vi "Sievert_auto.vi"() -> ()   [LabVIEW 2011]
uses:
  <vilib>/Utility/error.llb/DialogType.ctl
  <vilib>/DAQmx/write.llb/DAQmx Write (Digital Bool 1Line 1Point).vi
  <vilib>/Analysis/Matrix/Numeric/Conversions/Array To Matrix - RA.vi
  <vilib>/Analysis/Matrix/Numeric/Conversions/Matrix To Array - RM.vi
  <vilib>/DAQmx/create/channels.llb/DAQmx Create Channel (DO-Digital Output).vi
  <vilib>/DAQmx/miscellaneous.llb/DAQmx Fill In Error Info.vi
  <vilib>/Analysis/NI_AALPro.lvlib
  <vilib>/Analysis/Matrix/NI_Matrix.lvlib
  <vilib>/Analysis/NI_AALBase.lvlib
panel:
  in  "N fit patamar":i32=100
  in  "patamar milliseconds to wait":u32=500
  out "estagio 5":i32
  out "FIM":bool=TRUE
  out "limpo":i32
  in  "N fit":i32=5
  in  "Estagio auto":i32
  in  "ATM wait":u32
  in  "SET":i32
  in  "time subarray":dbl[](array[numeric])
  out "P cinetica mean 2":dbl format="%0.2f"
  out "T cinetica mean 3":dbl format="%0.2f"
  out "Time cinetica":dbl format="%0.2f"
  in  "T subarray 3":dbl[](array[numeric])
  in  "P T  index 2":i32
  in  "P subarray 2":dbl[](array[numeric])
  in  "Numeric":dbl=4.0
  in  "T subarray 2":dbl[](array[numeric])
  out "T cinetica mean 2":dbl format="%0.2f"
  out "P cinetica mean":dbl format="%0.2f"
  in  "P subarray":dbl[](array[numeric])
  in  "P T  index":i32
  out "T string":string
  out "P string":string
  out "path 2_cinetica":path
  out "Polynomial Coefficients 2":dbl[](array[numeric])
  out "Polynomial Coefficients":dbl[](array[numeric])
  in  "Count SET":i32=-1
  out "Set atual":i32
  out "mean pressure":dbl format="%.4p"
  out "Set number":i32
  in  "Tab Control":enum32{"Manual", "Automatico", "RLC - CDH2"}(tab)
  out "T":bool
  out "ZPf2":bool
  out "Pf2":bool
  out "Pit":bool
  out "ZPit":bool
  out "Camara":dbl(slide) scale=0.0..20.0 scale format="%#_3g"
  in  "Save manual":bool
  in  "Open Button":bool
  out "String 2":string
  in  "ATM":bool
  in  "Câmara":bool
  in  "Vácuo":bool
  in  "Entrada Gás":bool
  in  "Manual Ctrl":bool
  in  "stop":bool
  out "P-manual":dynamicdata(graph)
  in  "Clear":bool
  out "path":path
  in  "Nota":string
  in  "Sample name":string
  in  "File name":string
  out "Linear Model Graph":dbl[][](graph)
  out "Linear Model Graph 2":dbl[][](graph)
  in  "N to fit":i32=60
  out "N":i32
  out "Vácuo":bool
  out "Atm":bool
  out "Câmara":bool
  out "String_cinetica":string
  out "Vol Ref":dbl(slide) scale=0.0..50.0 scale format="%#_4f"
  out "Entrada gás":bool
  in  "Guardar\nCinetica":bool
  out "p fit":dbl format="%#_4g"
  out "T fit":dbl format="%#_4g"
  in  "Open Button 2":bool
  out "x >= y?":bool
  in  "seconds":dbl
  out "Elapsed Time (sec)":dbl format="%.1f"
  out "Boolean 3":bool
  out "String 3":string
  out "T 2":bool
  out "ZPit 2":bool
  out "Pit 2":bool
  out "Pf2 2":bool
  out "ZPf2 2":bool
  out "Camara 2":dbl(slide) scale=0.0..6.0 scale format="%#_3g"
  out "Vácuo 2":bool
  out "Atm 2":bool
  out "Câmara 2":bool
  out "Vol Ref 3":dbl(slide) scale=0.0..6.0 scale format="%#_4f"
  out "Entrada gás 2":bool
  in  "Auto Ctrl":bool
  in  "Play Button":bool
  out "time stamp":timestamp format="%<%.2X>T"
  out "Time (sec)":dbl format="%.1f"
  in  "clear":bool
  out "Automatico":dynamicdata(graph)
  out "Linear P":T1(graph)
  out "Linear T":T1(graph)
  out "Contador":i32
  in  "STOP Slope":dbl
  out "P slope":dbl
  out "slope":dbl format="%#_4g"
  out "P fit":dbl format="%#_4g"
  out "T fit":dbl format="%#_4g"
  out "x = y?":bool
  out "teste slope":i32
  in  "Set P auto":dbl
  in  "Step P":dbl=2.0
  in  "P_max":dbl=2.0
  in  "P_max camara":dbl=2.0
  out "Carga":bool=TRUE
  out "Descarga":bool
  out "String":string
  in  "P_min descarga":dbl
  in  "Boolean":bool
  in  "Array":dbl[](array[numeric])
  out "Boolean 2":bool
  out "Desc SET":i32
  in  "ZPf2 time":dbl=24.0
  in  "Ciclos":dbl
  out "Efetuados":dbl
  # "P vol ref"
  # "P Câmara"
  # "P vol ref"
  # "P Câmara"
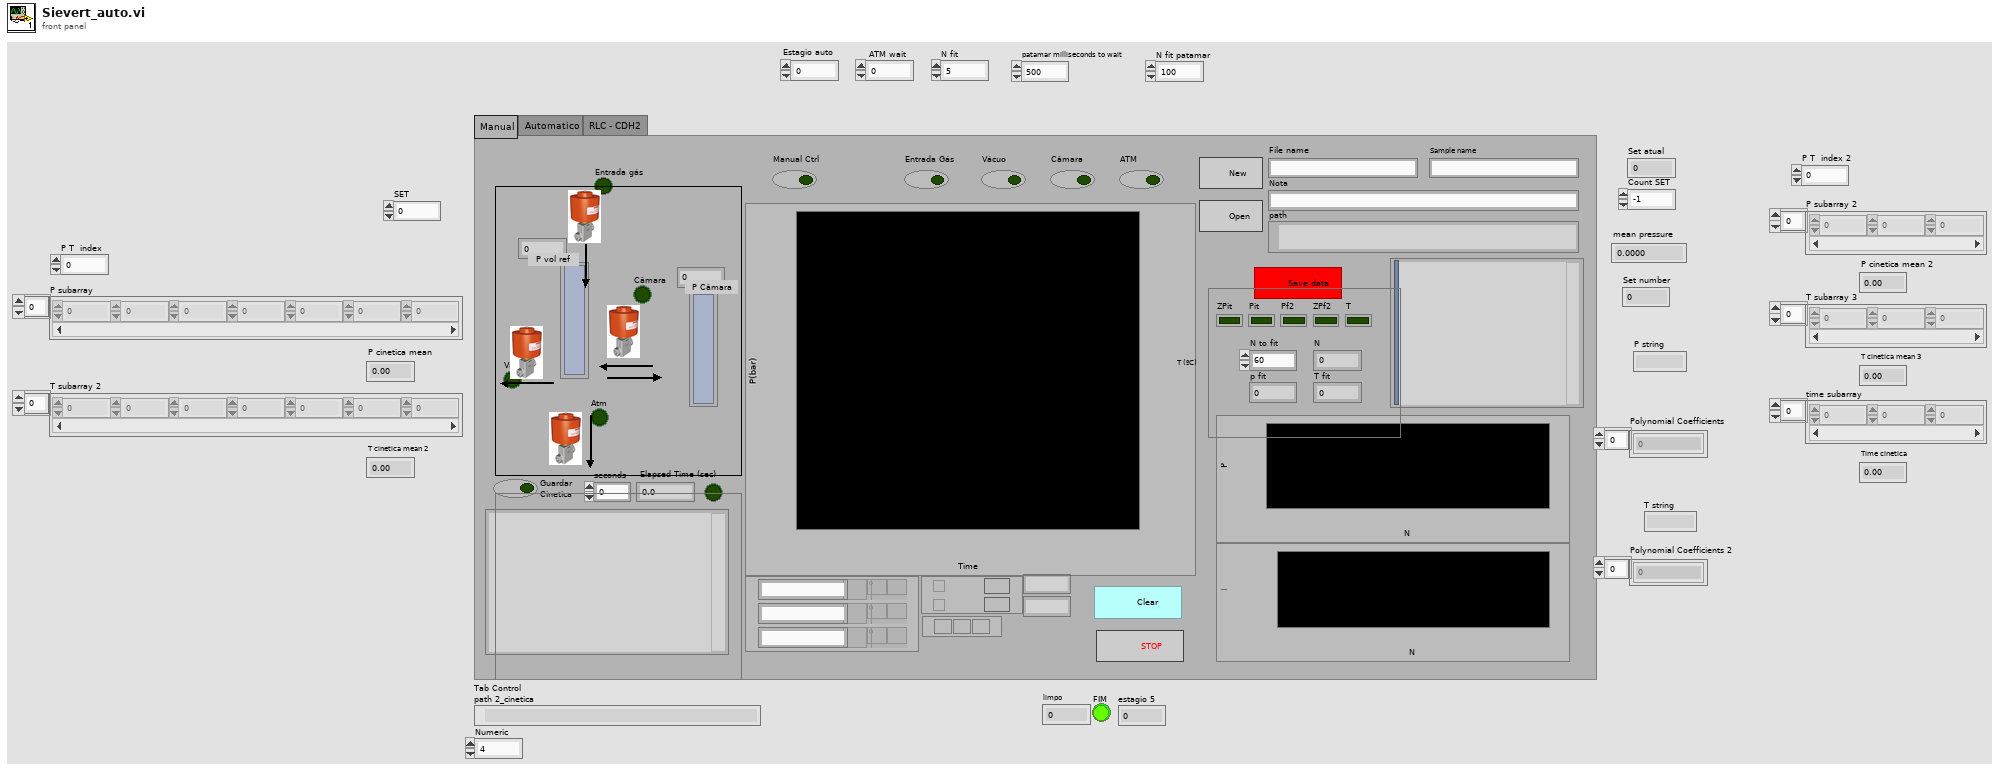
[diagram p1: front panel]
types:
  T1 = cluster{"Real 2D Array":dbl[], "Best Linear Fit":dbl[]}[]
  T2 = enum16{"open", "replace", "create", "open or create", "replace or create", "replace or create with confirmation"}
  T3 = typedef "NI_Matrix.lvlib/RealMatrix.ctl" = dbl[][]
  T4 = typedef "DialogType.ctl" = u16
  T5 = cluster{"Real 2D Array":dbl[], "Best Polynomial Fit":dbl[]}
  T6 = cluster{"Real 2D Array":dbl[], "Best Linear Fit":dbl[]}
  T7 = cluster{"Real 2D Array":dbl[], "Real 2D Array":dbl[]}
  T8 = cluster{"Real 2D Array":dbl[], "Best Polynomial Fit":dbl[]}[]
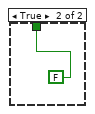
[diagram p2: hidden frame]
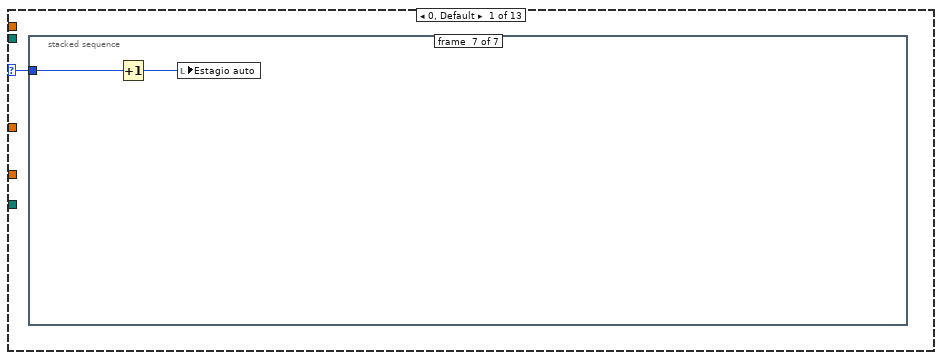
[diagram p5: hidden frame]
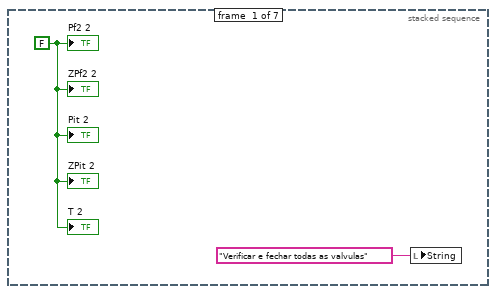
[diagram p6: hidden frame]
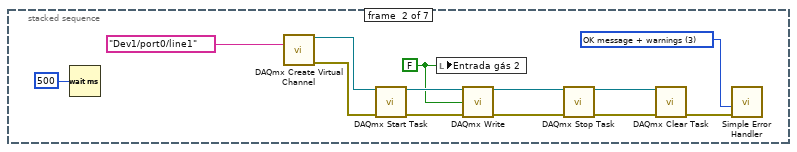
[diagram p7: hidden frame]
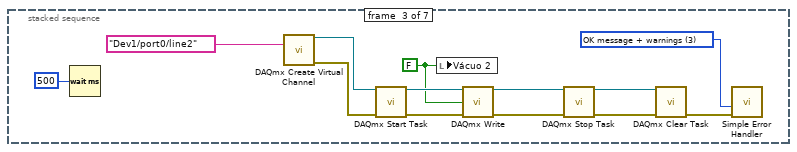
[diagram p8: hidden frame]
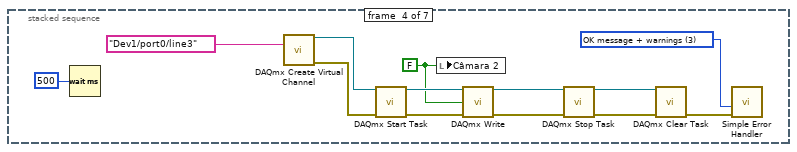
[diagram p9: hidden frame]
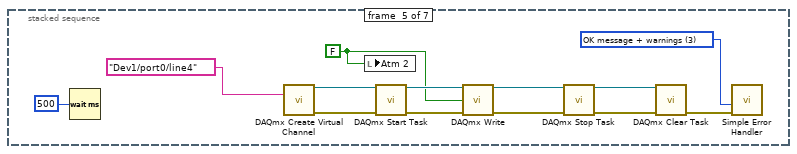
[diagram p10: hidden frame]
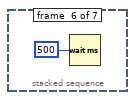
[diagram p11: hidden frame]
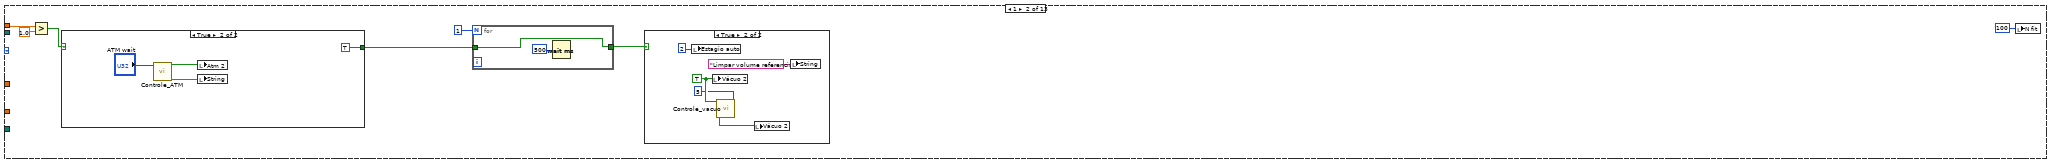
[diagram p12: hidden frame]
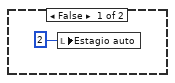
[diagram p13: hidden frame]
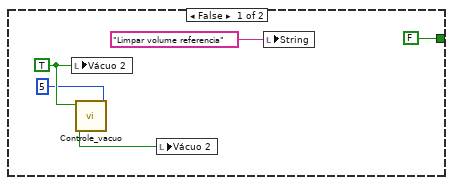
[diagram p14: hidden frame]
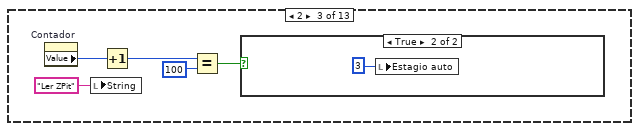
[diagram p15: hidden frame]
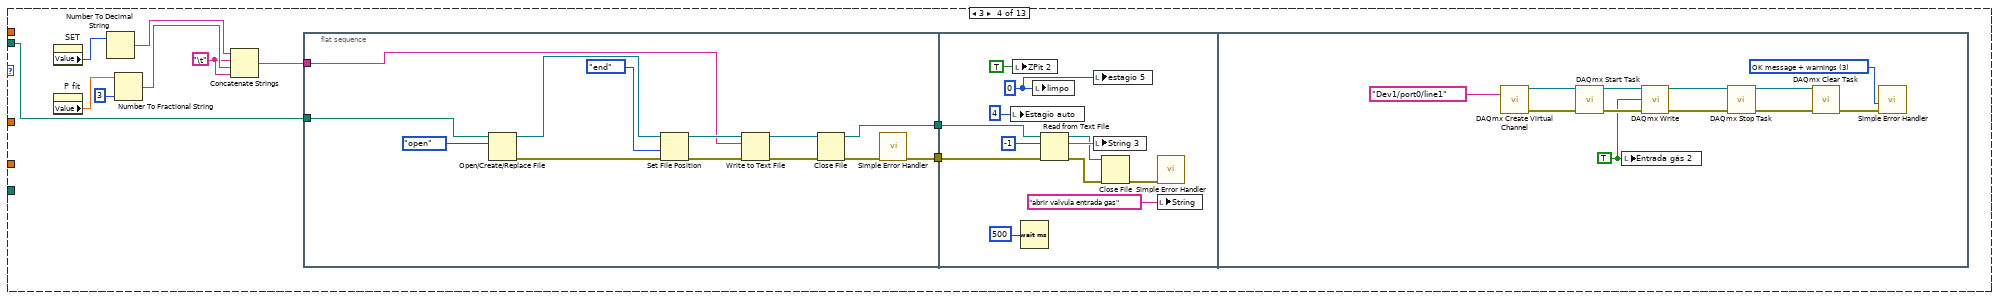
[diagram p17: hidden frame]
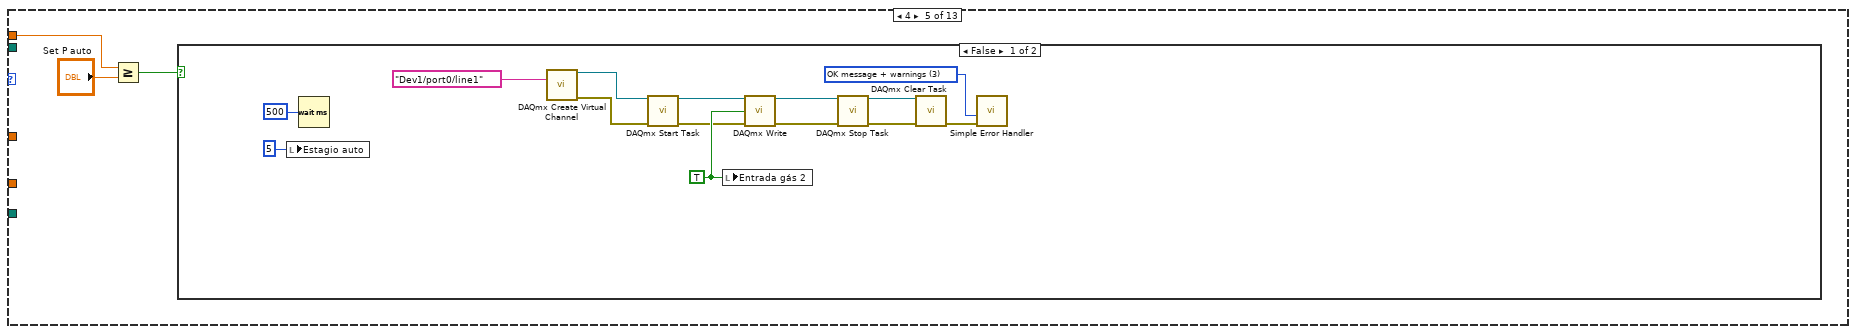
[diagram p18: hidden frame]
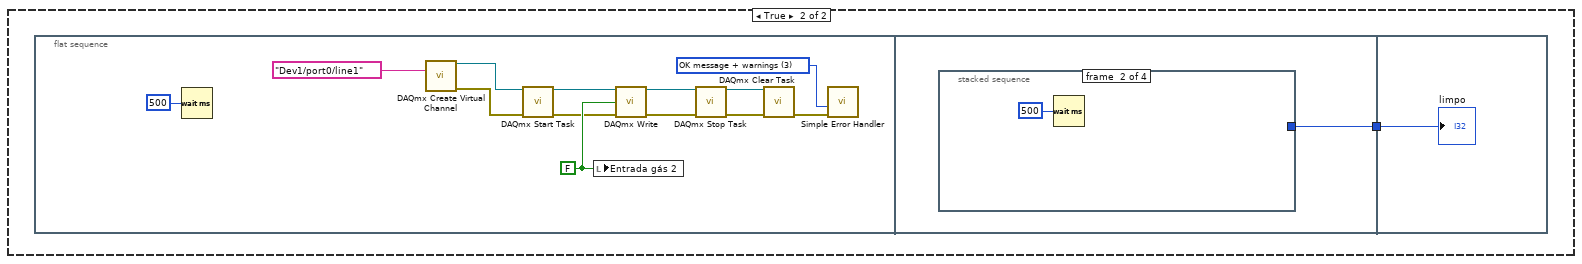
[diagram p19: hidden frame]
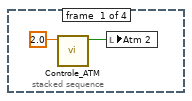
[diagram p20: hidden frame]
diagram:
  n1 = local write "P_min descarga"(0.025 ("P_min descarga")) -> ()
  n2 = local write "P_max camara"(25.0 ("P_max camara")) -> ()
  n3 = local write "Array"(dbl[] [0.5, 1.0, 2.0, 3.0, 4.0, 5.0, 6.0, 7.0, 8.0, 9.0, 10.0, 11.0, 12.0, 13.0, 14.0, 15.0, 16.0, 17.0, 18.0, 19.0, 20.0, 30.0, 40.0, 50.0, 60.0, 70.0] ("Array")) -> ()
  n4 = local write "Set P auto"(0.5 ("Set P auto")) -> ()
  n5 = local write "teste slope"(0 ("teste slope")) -> ()
  n6 = local write "Efetuados"(0.0 ("Efetuados")) -> ()
  n7 = local write "Desc SET"(0 ("Desc SET")) -> ()
  n8 = local write "P_max"(50.0 ("P_max")) -> ()
  n9 = local write "Ciclos"(0.0 ("Ciclos")) -> ()
  n10 = local write "Carga"(TRUE ("Carga")) -> ()
  n11 = local write "Descarga"(FALSE ("Descarga")) -> ()
  n12 = local write "estagio 5"(0 ("estagio 5")) -> ()
  n13 = local write "SET"(0 ("SET auto")) -> ()
  n14 = while {
    stop <- w28 stop-if-true
    n15 = case shown="False" "Auto Ctrl" {
      tunnel: [TRUE ("Auto Ctrl") FALSE ("Auto Ctrl")] -> w29
      frame False {
      }
      frame True {
      }
    }
    n16 = local write "Manual Ctrl"(w29) -> ()
    n17 = case shown="True" "Auto Ctrl" {
      frame False {
      }
      frame True {
        n18 = for {
          N: "N fit" -> [w50]
          i -> [w52]
          w56 = 0 ("polynomial order")
          w47 = 0 ("polynomial order")
          n19 = case shown="True" "clear" {
            frame False {
            }
            frame True {
              n20 = property on="Linear T" class="XYGraph (strict)"("Value"=T1 [] ("Linear T")) -> ()  [unwired: 2 in, 2 out]
              n21 = property on="Linear P" class="XYGraph (strict)"("Value"=T1 [] ("Linear P")) -> ()  [unwired: 2 in, 2 out]
              n22 = property on="Automatico" class="WFChart (strict)"("History Data"=dynamicdata[] []) -> ()  [unwired: 2 in, 2 out]
            }
          }
          n23 = Increment(x=w52) -> (x+1=w51:i32)
          n24 = Equal?(x=w51, y=w50) -> (x = y?=w53:bool)
          "x = y?" <- w53
          n25 = call "Elapsed Time2"("Reset"=w53) -> ("Elapsed Time (s)"=w67:dbl)  [unwired: 11 in, 7 out]
          "Time (sec)" <- w67
          n26 = call "Read P T.vi"() -> ("P Set 2 Output 2"=w77:dbl, "T Set 2 Output"=w46:dbl)  [unwired: 4 in, 6 out]
          n27 = Multiply(x=w77, y=10.0) -> (x*y=w45:dbl)
          n28 = stacked-sequence {
            tunnel: w45 -> [w713 _]
            tunnel: w46 -> [w699 _]
            tunnel: [w680 _] -> w65
            tunnel: [w696 _] -> w64
            tunnel: w67 -> [w683 _]
            tunnel: [w681 _] -> w61
            tunnel: [w679 _] -> w42
            tunnel: [w678 _] -> w41
            frame #0 {
              w682 = 2 ("y")
              n29 = property on="P subarray 2" class="Arr (strict)"() -> ("Value"=w715:dbl[])  [unwired: 2 in, 2 out]
              n30 = property on="T subarray 3" class="Arr (strict)"() -> ("Value"=w705:dbl[])  [unwired: 2 in, 2 out]
              n31 = property on="time subarray" class="Arr (strict)"() -> ("Value"=w692:dbl[])  [unwired: 2 in, 2 out]
              n32 = property on="P T  index 2" class="DigNum (strict)"() -> ("Value"=w684:i32)  [unwired: 2 in, 2 out]
              n33 = Replace Array Subset(array=w692, new element=w683, index=w684) -> (w685:dbl[])
              n34 = Replace Array Subset(array=w715, new element=w713, index=w684) -> (w698:dbl[])
              n35 = Replace Array Subset(array=w705, new element=w699, index=w684) -> (w697:dbl[])
              n36 = call-poly <vilib>:"Array To Matrix.vi"("Real 1D Array"=w685) -> ("Real Matrix (Column Vector)"=w695:T3)
              n37 = call-poly <vilib>:"Array To Matrix.vi"("Real 1D Array"=w698) -> ("Real Matrix (Column Vector)"=w718:T3)
              n38 = call-poly <vilib>:"Array To Matrix.vi"("Real 1D Array"=w697) -> ("Real Matrix (Column Vector)"=w708:T3)
              n39 = Matrix Size(0:w695) -> (1:w694:i32, 2:w693:i32)
              n40 = Matrix Size(0:w718) -> (1:w717:i32, 2:w716:i32)
              n41 = Matrix Size(0:w708) -> (1:w707:i32, 2:w706:i32)
              n42 = Increment(x=w694) -> (x+1=w686:i32)
              n43 = Increment(x=w717) -> (x+1=w709:i32)
              n44 = Increment(x=w707) -> (x+1=w700:i32)
              n45 = Resize Matrix(1:w693, 2:w686, 4:w695) -> (0:w691:T3)
              n46 = Resize Matrix(1:w716, 2:w709, 4:w718) -> (0:w714:T3)
              n47 = Resize Matrix(1:w706, 2:w700, 4:w708) -> (0:w704:T3)
              n48 = call-poly <vilib>:"Matrix To Array.vi"("Real Matrix"=w691) -> ("Real 2D Array"=w689:dbl[][])
              n49 = call-poly <vilib>:"Matrix To Array.vi"("Real Matrix"=w714) -> ("Real 2D Array"=w712:dbl[][])
              n50 = call-poly <vilib>:"Matrix To Array.vi"("Real Matrix"=w704) -> ("Real 2D Array"=w703:dbl[][])
              n51 = Subtract(x=w686, y=w682) -> (x-y=w687:i32)
              n52 = Subtract(x=w709, y=w682) -> (x-y=w710:i32)
              n53 = Subtract(x=w700, y=w682) -> (x-y=w701:i32)
              n54 = Reshape Array(w689, w686) -> (w688:dbl[])
              n55 = Reshape Array(w712, w709) -> (w711:dbl[])
              n56 = Reshape Array(w703, w700) -> (w702:dbl[])
              n57 = local write "time subarray"(w688) -> ()
              n58 = Reshape Array(w688, w687) -> (w681:dbl[])
              n59 = local write "P subarray 2"(w711) -> ()
              n60 = Reshape Array(w711, w710) -> (w680:dbl[])
              n61 = local write "T subarray 3"(w702) -> ()
              n62 = Reshape Array(w702, w701) -> (w696:dbl[])
              n63 = call <vilib>:"Mean.vi"("X"=w681) -> ("mean"=→"Time cinetica":dbl)  [unwired: 1 out]
              n64 = call <vilib>:"Mean.vi"("X"=w680) -> ("mean"=w679:dbl)  [unwired: 1 out]
              "P cinetica mean 2" <- w679
              n65 = call <vilib>:"Mean.vi"("X"=w696) -> ("mean"=w678:dbl)  [unwired: 1 out]
              "T cinetica mean 3" <- w678
            }
            frame #1 {
              n66 = property on="P T  index 2" class="DigNum (strict)"() -> ("Value"=w720:i32)  [unwired: 2 in, 2 out]
              n67 = Increment(x=w720) -> (x+1=w719:i32)
              n68 = local write "P T  index 2"(w719) -> ()
            }
          }
          n69 = local write "Vol Ref 3"(w45) -> ()
          n70 = Merge Signals(w45, w46) -> (→"Automatico":dynamicdata)
          n71 = To Time Stamp(1:w67) -> (0:→"time stamp":timestamp)
          n72 = property on="path 2_cinetica" class="Path"() -> ("Value"=w43:path)  [unwired: 2 in, 2 out]
          n73 = call <vilib>:"Linear Fit.vi"("Y"=w64, "X"=w61) -> ("Best Linear Fit"=w73:dbl[])  [unwired: 9 in, 4 out]
          n74 = call <vilib>:"General Polynomial Fit.vi"("Y"=w65, "polynomial order"=w47, "X"=w61) -> ("Best Polynomial Fit"=w63:dbl[], "Polynomial Coefficients"=w58:dbl[])  [unwired: 9 in, 2 out]
          n75 = call <vilib>:"General Polynomial Fit.vi"("Y"=w64, "polynomial order"=w47, "X"=w61) -> ("Best Polynomial Fit"=w62:dbl[], "Polynomial Coefficients"=w57:dbl[])  [unwired: 9 in, 2 out]
          n76 = call <vilib>:"Linear Fit.vi"("Y"=w65, "X"=w61) -> ("Best Linear Fit"=w68:dbl[], "slope"=w48:dbl)  [unwired: 9 in, 3 out]
          "slope" <- w48
          n77 = property on="path" class="Path"() -> ("Value"=w44:path)  [unwired: 2 in, 2 out]
          n78 = case shown="True" "Play Button" {
            tunnel: w44 -> [_ w84]
            tunnel: w45 -> [_ w83]
            tunnel: w43 -> [_ w82]
            tunnel: w42 -> [_ w81]
            tunnel: w41 -> [_ w80]
            frame False {
            }
            frame True {
              n79 = case shown="9" "Estagio auto" {
                selector: "Estagio auto" -> [w86 _ _ _ _ _ _ _ _ _ _ _ _]
                tunnel: w84 -> [_ _ _ w175 _ _ w318 _ w434 _ _ w509 w595]
                tunnel: w83 -> [_ w144 _ _ w221 w265 _ _ _ w468 _ _ _]
                tunnel: w82 -> [_ _ _ _ _ _ _ w356 _ _ _ _ _]
                tunnel: w81 -> [_ _ _ _ _ _ _ w355 _ _ _ _ _]
                tunnel: w80 -> [_ _ _ _ _ _ _ w354 _ _ _ _ _]
                frame 0, Default {
                  n80 = stacked-sequence {
                    tunnel: w86 -> [_ _ _ _ _ _ w142]
                    frame #0 {
                      w87 = FALSE ("Pit")
                      n81 = local write "String"("Verificar e fechar todas as valvulas" ("String")) -> ()
                      "ZPf2 2" <- w87
                      "Pf2 2" <- w87
                      "Pit 2" <- w87
                      "ZPit 2" <- w87
                      "T 2" <- w87
                    }
                    frame #1 {
                      w90 = FALSE ("Boolean 4")
                      w95 = T4 3 items=["no dialog", "OK message", "continue or stop message", "OK message + warnings", "continue/stop + warnings"] ("type of dialog (OK msg:1)")
                      n82 = Wait (ms)(milliseconds to wait=u32 500) -> ()  [unwired: 1 out]
                      n83 = call-poly <vilib>:"DAQmx Create Virtual Channel.vi"("lines"=tag "Dev1/port0/line1") -> ("task out"=w93:refnum<k21>, "error out"=w94:errorcluster)  [unwired: 13 in]
                      n84 = call <vilib>:"DAQmx Start Task.vi"("task/channels in"=w93, "error in"=w94) -> ("task out"=w96:refnum<k21>, "error out"=w97:errorcluster)  [unwired: 12 in]
                      n85 = local write "Entrada gás 2"(w90) -> ()
                      n86 = call-poly <vilib>:"DAQmx Write.vi"("task/channels in"=w96, "data"=w90, "error in"=w97) -> ("task out"=w101:refnum<k21>, "error out"=w98:errorcluster)  [unwired: 10 in, 1 out]
                      n87 = call <vilib>:"DAQmx Stop Task.vi"("task/channels in"=w101, "error in"=w98) -> ("task out"=w100:refnum<k21>, "error out"=w99:errorcluster)  [unwired: 12 in]
                      n88 = call <vilib>:"DAQmx Clear Task.vi"("task in"=w100, "error in"=w99) -> ("error out"=w92:errorcluster)  [unwired: 13 in]
                      n89 = call <vilib>:"Simple Error Handler.vi"("type of dialog (OK msg:1)"=w95, "error in (no error)"=w92) -> ()  [unwired: 3 in, 5 out]
                    }
                    frame #2 {
                      w103 = FALSE ("Boolean 4")
                      w108 = T4 3 items=["no dialog", "OK message", "continue or stop message", "OK message + warnings", "continue/stop + warnings"] ("type of dialog (OK msg:1)")
                      n90 = Wait (ms)(milliseconds to wait=u32 500) -> ()  [unwired: 1 out]
                      n91 = call-poly <vilib>:"DAQmx Create Virtual Channel.vi"("lines"=tag "Dev1/port0/line2") -> ("task out"=w106:refnum<k21>, "error out"=w107:errorcluster)  [unwired: 13 in]
                      n92 = call <vilib>:"DAQmx Start Task.vi"("task/channels in"=w106, "error in"=w107) -> ("task out"=w109:refnum<k21>, "error out"=w110:errorcluster)  [unwired: 12 in]
                      n93 = local write "Vácuo 2"(w103) -> ()
                      n94 = call-poly <vilib>:"DAQmx Write.vi"("task/channels in"=w109, "data"=w103, "error in"=w110) -> ("task out"=w114:refnum<k21>, "error out"=w111:errorcluster)  [unwired: 10 in, 1 out]
                      n95 = call <vilib>:"DAQmx Stop Task.vi"("task/channels in"=w114, "error in"=w111) -> ("task out"=w113:refnum<k21>, "error out"=w112:errorcluster)  [unwired: 12 in]
                      n96 = call <vilib>:"DAQmx Clear Task.vi"("task in"=w113, "error in"=w112) -> ("error out"=w105:errorcluster)  [unwired: 13 in]
                      n97 = call <vilib>:"Simple Error Handler.vi"("type of dialog (OK msg:1)"=w108, "error in (no error)"=w105) -> ()  [unwired: 3 in, 5 out]
                    }
                    frame #3 {
                      w116 = FALSE ("Boolean 4")
                      w121 = T4 3 items=["no dialog", "OK message", "continue or stop message", "OK message + warnings", "continue/stop + warnings"] ("type of dialog (OK msg:1)")
                      n98 = Wait (ms)(milliseconds to wait=u32 500) -> ()  [unwired: 1 out]
                      n99 = call-poly <vilib>:"DAQmx Create Virtual Channel.vi"("lines"=tag "Dev1/port0/line3") -> ("task out"=w119:refnum<k21>, "error out"=w120:errorcluster)  [unwired: 13 in]
                      n100 = call <vilib>:"DAQmx Start Task.vi"("task/channels in"=w119, "error in"=w120) -> ("task out"=w122:refnum<k21>, "error out"=w123:errorcluster)  [unwired: 12 in]
                      n101 = local write "Câmara 2"(w116) -> ()
                      n102 = call-poly <vilib>:"DAQmx Write.vi"("task/channels in"=w122, "data"=w116, "error in"=w123) -> ("task out"=w127:refnum<k21>, "error out"=w124:errorcluster)  [unwired: 10 in, 1 out]
                      n103 = call <vilib>:"DAQmx Stop Task.vi"("task/channels in"=w127, "error in"=w124) -> ("task out"=w126:refnum<k21>, "error out"=w125:errorcluster)  [unwired: 12 in]
                      n104 = call <vilib>:"DAQmx Clear Task.vi"("task in"=w126, "error in"=w125) -> ("error out"=w118:errorcluster)  [unwired: 13 in]
                      n105 = call <vilib>:"Simple Error Handler.vi"("type of dialog (OK msg:1)"=w121, "error in (no error)"=w118) -> ()  [unwired: 3 in, 5 out]
                    }
                    frame #4 {
                      w129 = FALSE ("Boolean 4")
                      w134 = T4 3 items=["no dialog", "OK message", "continue or stop message", "OK message + warnings", "continue/stop + warnings"] ("type of dialog (OK msg:1)")
                      n106 = Wait (ms)(milliseconds to wait=u32 500) -> ()  [unwired: 1 out]
                      n107 = call-poly <vilib>:"DAQmx Create Virtual Channel.vi"("lines"=tag "Dev1/port0/line4") -> ("task out"=w132:refnum<k21>, "error out"=w133:errorcluster)  [unwired: 13 in]
                      n108 = local write "Atm 2"(w129) -> ()
                      n109 = call <vilib>:"DAQmx Start Task.vi"("task/channels in"=w132, "error in"=w133) -> ("task out"=w135:refnum<k21>, "error out"=w136:errorcluster)  [unwired: 12 in]
                      n110 = call-poly <vilib>:"DAQmx Write.vi"("task/channels in"=w135, "data"=w129, "error in"=w136) -> ("task out"=w140:refnum<k21>, "error out"=w137:errorcluster)  [unwired: 10 in, 1 out]
                      n111 = call <vilib>:"DAQmx Stop Task.vi"("task/channels in"=w140, "error in"=w137) -> ("task out"=w139:refnum<k21>, "error out"=w138:errorcluster)  [unwired: 12 in]
                      n112 = call <vilib>:"DAQmx Clear Task.vi"("task in"=w139, "error in"=w138) -> ("error out"=w131:errorcluster)  [unwired: 13 in]
                      n113 = call <vilib>:"Simple Error Handler.vi"("type of dialog (OK msg:1)"=w134, "error in (no error)"=w131) -> ()  [unwired: 3 in, 5 out]
                    }
                    frame #5 {
                      n114 = Wait (ms)(milliseconds to wait=u32 500) -> ()  [unwired: 1 out]
                    }
                    frame #6 {
                      n115 = Increment(x=w142) -> (x+1=w143:i32)
                      n116 = local write "Estagio auto"(w143) -> ()
                    }
                  }
                }
                frame 1 {
                  n117 = Greater?(x=w144, y=1.0) -> (0:w150:bool)
                  n118 = case shown="True" w150 {
                    tunnel: [FALSE ("Boolean") TRUE ("Boolean")] -> w147
                    frame False {
                      w162 = TRUE ("Boolean")
                      n119 = local write "Vácuo 2"(w162) -> ()
                      n120 = call "Controle_vacuo.vi"("time (s) to wait vacuo"=u32 5, "Boolean"=w162) -> ("Vacuo"=w163:bool)  [unwired: 9 in]
                      n121 = local write "Vácuo 2"(w163) -> ()
                      n122 = local write "String"("Limpar volume referencia" ("String")) -> ()
                    }
                    frame True {
                      n123 = call "Controle_ATM.vi"("seconds to wait"="ATM wait") -> ("String 2"=w167:string, "Atm"=w166:bool)  [unwired: 9 in]
                      n124 = local write "Atm 2"(w166) -> ()
                      n125 = local write "String"(w167) -> ()
                    }
                  }
                  n126 = for {
                    N: 1 -> [_]
                    tunnel: [w152] -> w148
                    tunnel: w147 -> [w152]
                    n127 = Wait (ms)(milliseconds to wait=u32 500 ("x")) -> ()  [unwired: 1 out]
                  }
                  n128 = case shown="True" w148 {
                    frame False {
                      n129 = local write "Estagio auto"(2 ("Estagio auto")) -> ()
                    }
                    frame True {
                      w157 = TRUE ("Boolean")
                      n130 = local write "Estagio auto"(2 ("Estagio auto")) -> ()
                      n131 = local write "Vácuo 2"(w157) -> ()
                      n132 = call "Controle_vacuo.vi"("time (s) to wait vacuo"=u32 5, "Boolean"=w157) -> ("Vacuo"=w158:bool)  [unwired: 9 in]
                      n133 = local write "Vácuo 2"(w158) -> ()
                      n134 = local write "String"("Limpar volume referencia" ("String")) -> ()
                    }
                  }
                  n135 = local write "N fit"(100 ("N fit")) -> ()
                }
                frame 2 {
                  n136 = property on="Contador" class="DigNum (strict)"() -> ("Value"=w171:i32)  [unwired: 2 in, 2 out]
                  n137 = local write "String"("Ler ZPit" ("String")) -> ()
                  n138 = Increment(x=w171) -> (x+1=w170:i32)
                  n139 = Equal?(x=w170, y=100) -> (x = y?=w168:bool)
                  n140 = case shown="True" w168 {
                    frame False {
                    }
                    frame True {
                      n141 = local write "Estagio auto"(3 ("Estagio auto")) -> ()
                    }
                  }
                }
                frame 3 {
                  w180 = "\t"
                  n142 = property on="SET" class="DigNum (strict)"() -> ("Value"=w174:i32)  [unwired: 2 in, 2 out]
                  n143 = property on="P fit" class="DigNum (strict)"() -> ("Value"=w177:dbl)  [unwired: 2 in, 2 out]
                  n144 = Number To Decimal String(number=w174) -> (decimal integer string=w179:string)  [unwired: 1 in]
                  n145 = Number To Fractional String(number=w177, precision (6)=i16 3) -> (F-format string=w181:string)  [unwired: 2 in]
                  n146 = Concatenate Strings(w179, w180, w181, w180) -> (w178:string)
                  n147 = flat-sequence {
                    tunnel: [w187] -> w183
                    tunnel: [w186] -> w182
                    tunnel: w178 -> [w185]
                    tunnel: w175 -> [w184]
                    tunnel: w183 -> [w203]
                    tunnel: w182 -> [w202]
                    frame #0 {
                      n148 = Open/Create/Replace File(file path (use dialog)=w184, operation (0:open)=T2."open") -> (refnum out=w193:refnum<file>, error out=w194:errorcluster)  [unwired: 2 in, 3 out]
                      n149 = Set File Position(refnum=w193, from (0:start)=enum16{"start", "end", "current"}."end", error in=w194) -> (refnum out=w191:refnum<file>, error out=w190:errorcluster)  [unwired: 1 in]
                      n150 = Write to Text File(file (use dialog)=w191, text=w185, error in=w190) -> (refnum out=w195:refnum<file>, error out=w196:errorcluster)  [unwired: 2 out]
                      n151 = Close File(refnum=w195, error in=w196) -> (path=w187:path, error out=w188:errorcluster)
                      n152 = call <vilib>:"Simple Error Handler.vi"("error in (no error)"=w188) -> ("error out"=w186:errorcluster)  [unwired: 1 in, 7 out]
                    }
                    frame #1 {
                      w197 = 0 ("limpo")
                      n153 = local write "Estagio auto"(4 ("Estagio auto")) -> ()
                      n154 = local write "ZPit 2"(TRUE ("ZPit")) -> ()
                      n155 = Wait (ms)(milliseconds to wait=u32 500) -> ()  [unwired: 1 out]
                      n156 = local write "limpo"(w197) -> ()
                      n157 = Read from Text File(file (use dialog)=w203, count=-1 ("Count  3"), error in=w202) -> (refnum out=w204:refnum<file>, text=w208:string, error out=w205:errorcluster)  [unwired: 1 in, 1 out]
                      n158 = local write "estagio 5"(w197) -> ()
                      n159 = local write "String 3"(w208) -> ()
                      n160 = Close File(refnum=w204, error in=w205) -> (error out=w206:errorcluster)  [unwired: 1 out]
                      n161 = call <vilib>:"Simple Error Handler.vi"("error in (no error)"=w206) -> ()  [unwired: 1 in, 8 out]
                      n162 = local write "String"("abrir valvula entrada gas" ("String")) -> ()
                    }
                    frame #2 {
                      w209 = T4 3 items=["no dialog", "OK message", "continue or stop message", "OK message + warnings", "continue/stop + warnings"] ("type of dialog (OK msg:1)")
                      w215 = TRUE ("Boolean 4")
                      n163 = call-poly <vilib>:"DAQmx Create Virtual Channel.vi"("lines"=tag "Dev1/port0/line1") -> ("task out"=w217:refnum<k21>, "error out"=w218:errorcluster)  [unwired: 13 in]
                      n164 = call <vilib>:"DAQmx Start Task.vi"("task/channels in"=w217, "error in"=w218) -> ("task out"=w219:refnum<k21>, "error out"=w220:errorcluster)  [unwired: 12 in]
                      n165 = local write "Entrada gás 2"(w215) -> ()
                      n166 = call-poly <vilib>:"DAQmx Write.vi"("task/channels in"=w219, "data"=w215, "error in"=w220) -> ("task out"=w212:refnum<k21>, "error out"=w211:errorcluster)  [unwired: 10 in, 1 out]
                      n167 = call <vilib>:"DAQmx Stop Task.vi"("task/channels in"=w212, "error in"=w211) -> ("task out"=w213:refnum<k21>, "error out"=w214:errorcluster)  [unwired: 12 in]
                      n168 = call <vilib>:"DAQmx Clear Task.vi"("task in"=w213, "error in"=w214) -> ("error out"=w210:errorcluster)  [unwired: 13 in]
                      n169 = call <vilib>:"Simple Error Handler.vi"("type of dialog (OK msg:1)"=w209, "error in (no error)"=w210) -> ()  [unwired: 3 in, 5 out]
                    }
                  }
                }
                frame 4 {
                  n170 = Greater Or Equal?(x=w221, y="Set P auto") -> (x >= y?=w223:bool)
                  n171 = case shown="False" w223 {
                    frame False {
                      w231 = T4 3 items=["no dialog", "OK message", "continue or stop message", "OK message + warnings", "continue/stop + warnings"] ("type of dialog (OK msg:1)")
                      w237 = TRUE ("data")
                      n172 = local write "Estagio auto"(5 ("Estagio auto")) -> ()
                      n173 = Wait (ms)(milliseconds to wait=u32 500) -> ()  [unwired: 1 out]
                      n174 = call-poly <vilib>:"DAQmx Create Virtual Channel.vi"("lines"=tag "Dev1/port0/line1") -> ("task out"=w228:refnum<k21>, "error out"=w227:errorcluster)  [unwired: 13 in]
                      n175 = call <vilib>:"DAQmx Start Task.vi"("task/channels in"=w228, "error in"=w227) -> ("task out"=w226:refnum<k21>, "error out"=w225:errorcluster)  [unwired: 12 in]
                      n176 = local write "Entrada gás 2"(w237) -> ()
                      n177 = call-poly <vilib>:"DAQmx Write.vi"("task/channels in"=w226, "data"=w237, "error in"=w225) -> ("task out"=w234:refnum<k21>, "error out"=w233:errorcluster)  [unwired: 10 in, 1 out]
                      n178 = call <vilib>:"DAQmx Stop Task.vi"("task/channels in"=w234, "error in"=w233) -> ("task out"=w236:refnum<k21>, "error out"=w235:errorcluster)  [unwired: 12 in]
                      n179 = call <vilib>:"DAQmx Clear Task.vi"("task in"=w236, "error in"=w235) -> ("error out"=w232:errorcluster)  [unwired: 13 in]
                      n180 = call <vilib>:"Simple Error Handler.vi"("type of dialog (OK msg:1)"=w231, "error in (no error)"=w232) -> ()  [unwired: 3 in, 5 out]
                    }
                    frame True {
                      n181 = flat-sequence {
                        tunnel: [w252] -> w238
                        tunnel: w238 -> [w262]
                        frame #0 {
                          w244 = T4 3 items=["no dialog", "OK message", "continue or stop message", "OK message + warnings", "continue/stop + warnings"] ("type of dialog (OK msg:1)")
                          w251 = FALSE ("data")
                          n182 = Wait (ms)(milliseconds to wait=u32 500) -> ()  [unwired: 1 out]
                          n183 = call-poly <vilib>:"DAQmx Create Virtual Channel.vi"("lines"=tag "Dev1/port0/line1") -> ("task out"=w242:refnum<k21>, "error out"=w243:errorcluster)  [unwired: 13 in]
                          n184 = call <vilib>:"DAQmx Start Task.vi"("task/channels in"=w242, "error in"=w243) -> ("task out"=w240:refnum<k21>, "error out"=w239:errorcluster)  [unwired: 12 in]
                          n185 = local write "Entrada gás 2"(w251) -> ()
                          n186 = call-poly <vilib>:"DAQmx Write.vi"("task/channels in"=w240, "data"=w251, "error in"=w239) -> ("task out"=w248:refnum<k21>, "error out"=w247:errorcluster)  [unwired: 10 in, 1 out]
                          n187 = call <vilib>:"DAQmx Stop Task.vi"("task/channels in"=w248, "error in"=w247) -> ("task out"=w250:refnum<k21>, "error out"=w249:errorcluster)  [unwired: 12 in]
                          n188 = call <vilib>:"DAQmx Clear Task.vi"("task in"=w250, "error in"=w249) -> ("error out"=w245:errorcluster)  [unwired: 13 in]
                          n189 = call <vilib>:"Simple Error Handler.vi"("type of dialog (OK msg:1)"=w244, "error in (no error)"=w245) -> ()  [unwired: 3 in, 5 out]
                        }
                        frame #1 {
                          n190 = stacked-sequence {
                            tunnel: [_ _ _ w259] -> w252
                            frame #0 {
                              n191 = call "Controle_ATM.vi"("seconds to wait"=2.0) -> ("Atm"=w254:bool)  [unwired: 9 in, 1 out]
                              n192 = local write "Atm 2"(w254) -> ()
                            }
                            frame #1 {
                              n193 = Wait (ms)(milliseconds to wait=u32 500) -> ()  [unwired: 1 out]
                            }
                            frame #2 {
                              w257 = TRUE ("Vácuo")
                              n194 = local write "Vácuo 2"(w257) -> ()
                              n195 = call "Controle_vacuo.vi"("time (s) to wait vacuo"=4.0, "Boolean"=w257) -> ("Vacuo"=w258:bool)  [unwired: 9 in]
                              n196 = local write "Vácuo 2"(w258) -> ()
                            }
                            frame #3 {
                              n197 = Wait (ms)(milliseconds to wait=u32 500) -> ()  [unwired: 1 out]
                              n198 = property on="limpo" class="DigNum (strict)"() -> ("Value"=w260:i32)  [unwired: 2 in, 2 out]
                              n199 = Increment(x=w260) -> (x+1=w259:i32)
                            }
                          }
                        }
                        frame #2 {
                          "limpo" <- w262
                        }
                      }
                    }
                  }
                }
                frame 5 {
                  n200 = property on="Set P auto" class="DigNum (strict)"() -> ("Value"=w264:dbl)  [unwired: 2 in, 2 out]
                  n201 = Greater Or Equal?(x=w265, y=w264) -> (x >= y?=w263:bool)
                  n202 = case shown="True" w263 {
                    selector: w263 -> [_ w287]
                    frame False {
                      n203 = flat-sequence {
                        tunnel: [w267] -> w266
                        tunnel: w266 -> [w283]
                        frame #0 {
                          w270 = T4 3 items=["no dialog", "OK message", "continue or stop message", "OK message + warnings", "continue/stop + warnings"] ("type of dialog (OK msg:1)")
                          w280 = TRUE ("Boolean 4")
                          n204 = call-poly <vilib>:"DAQmx Create Virtual Channel.vi"("lines"=tag "Dev1/port0/line1") -> ("task out"=w274:refnum<k21>, "error out"=w273:errorcluster)  [unwired: 13 in]
                          n205 = call <vilib>:"DAQmx Start Task.vi"("task/channels in"=w274, "error in"=w273) -> ("task out"=w272:refnum<k21>, "error out"=w271:errorcluster)  [unwired: 12 in]
                          n206 = local write "Entrada gás 2"(w280) -> ()
                          n207 = call-poly <vilib>:"DAQmx Write.vi"("task/channels in"=w272, "data"=w280, "error in"=w271) -> ("task out"=w277:refnum<k21>, "error out"=w276:errorcluster)  [unwired: 10 in, 1 out]
                          n208 = call <vilib>:"DAQmx Stop Task.vi"("task/channels in"=w277, "error in"=w276) -> ("task out"=w278:refnum<k21>, "error out"=w279:errorcluster)  [unwired: 12 in]
                          n209 = call <vilib>:"DAQmx Clear Task.vi"("task in"=w278, "error in"=w279) -> ("error out"=w269:errorcluster)  [unwired: 13 in]
                          n210 = property on="estagio 5" class="DigNum (strict)"() -> ("Value"=w268:i32)  [unwired: 2 in, 2 out]
                          n211 = call <vilib>:"Simple Error Handler.vi"("type of dialog (OK msg:1)"=w270, "error in (no error)"=w269) -> ()  [unwired: 3 in, 5 out]
                          n212 = Increment(x=w268) -> (x+1=w267:i32)
                        }
                        frame #1 {
                          n213 = Less?(x=w283, y=6) -> (x < y?=w281:bool)
                          n214 = case shown="False" w281 {
                            frame False {
                              n215 = local write "Estagio auto"(5 ("Estagio auto")) -> ()
                            }
                            frame True {
                              n216 = local write "Estagio auto"(4 ("Estagio auto")) -> ()
                            }
                          }
                          "estagio 5" <- w283
                        }
                      }
                    }
                    frame True {
                      n217 = flat-sequence {
                        tunnel: w287 -> [w288]
                        tunnel: [w288] -> w286
                        tunnel: w286 -> [w304]
                        frame #0 {
                          w289 = FALSE ("Boolean 4")
                          w294 = T4 3 items=["no dialog", "OK message", "continue or stop message", "OK message + warnings", "continue/stop + warnings"] ("type of dialog (OK msg:1)")
                          n218 = call-poly <vilib>:"DAQmx Create Virtual Channel.vi"("lines"=tag "Dev1/port0/line1") -> ("task out"=w292:refnum<k21>, "error out"=w293:errorcluster)  [unwired: 13 in]
                          n219 = call <vilib>:"DAQmx Start Task.vi"("task/channels in"=w292, "error in"=w293) -> ("task out"=w295:refnum<k21>, "error out"=w296:errorcluster)  [unwired: 12 in]
                          n220 = local write "Entrada gás 2"(w289) -> ()
                          n221 = call-poly <vilib>:"DAQmx Write.vi"("task/channels in"=w295, "data"=w289, "error in"=w296) -> ("task out"=w300:refnum<k21>, "error out"=w297:errorcluster)  [unwired: 10 in, 1 out]
                          n222 = call <vilib>:"DAQmx Stop Task.vi"("task/channels in"=w300, "error in"=w297) -> ("task out"=w299:refnum<k21>, "error out"=w298:errorcluster)  [unwired: 12 in]
                          n223 = call <vilib>:"DAQmx Clear Task.vi"("task in"=w299, "error in"=w298) -> ("error out"=w291:errorcluster)  [unwired: 13 in]
                          n224 = call <vilib>:"Simple Error Handler.vi"("type of dialog (OK msg:1)"=w294, "error in (no error)"=w291) -> ()  [unwired: 3 in, 5 out]
                        }
                        frame #1 {
                          n225 = property on="estagio 5" class="DigNum (strict)"() -> ("Value"=w302:i32)  [unwired: 2 in, 2 out]
                          n226 = Greater?(x=w302, y=5) -> (0:w305:bool)
                          n227 = And(x=w304, y=w305) -> (x .and. y?=w303:bool)
                          n228 = case shown="False" w303 {
                            frame False {
                              n229 = local write "Estagio auto"(4 ("Estagio auto")) -> ()
                              n230 = Wait (ms)(milliseconds to wait=u32 500) -> ()  [unwired: 1 out]
                            }
                            frame True {
                              n231 = property on="Contador" class="DigNum (strict)"() -> ("Value"=w308:i32)  [unwired: 2 in, 2 out]
                              n232 = local write "String"("Ler Pit" ("String")) -> ()
                              n233 = Increment(x=w308) -> (x+1=w311:i32)
                              n234 = Equal?(x=w311, y=100) -> (x = y?=w309:bool)
                              n235 = case shown="True" w309 {
                                frame False {
                                }
                                frame True {
                                n236 = local write "Estagio auto"(6 ("Estagio auto")) -> ()
                                }
                              }
                            }
                          }
                        }
                      }
                    }
                  }
                }
                frame 6 {
                  n237 = property on="Contador" class="DigNum (strict)"() -> ("Value"=w314:i32)  [unwired: 2 in, 2 out]
                  n238 = Increment(x=w314) -> (x+1=w317:i32)
                  n239 = Equal?(x=w317, y=100) -> (x = y?=w315:bool)
                  n240 = case shown="True" w315 {
                    tunnel: w318 -> [_ w319]
                    frame False {
                    }
                    frame True {
                      n241 = property on="P fit" class="DigNum (strict)"() -> ("Value"=w320:dbl)  [unwired: 2 in, 2 out]
                      n242 = Number To Fractional String(number=w320, precision (6)=i16 3) -> (F-format string=w324:string)  [unwired: 2 in]
                      n243 = Concatenate Strings(w324, "\t") -> (w322:string)
                      n244 = flat-sequence {
                        tunnel: [w330] -> w326
                        tunnel: [w329] -> w325
                        tunnel: w322 -> [w328]
                        tunnel: w319 -> [w327]
                        tunnel: w326 -> [w347]
                        tunnel: w325 -> [w346]
                        frame #0 {
                          n245 = Open/Create/Replace File(file path (use dialog)=w327, operation (0:open)=T2."open") -> (refnum out=w336:refnum<file>, error out=w337:errorcluster)  [unwired: 2 in, 3 out]
                          n246 = Set File Position(refnum=w336, from (0:start)=enum16{"start", "end", "current"}."end", error in=w337) -> (refnum out=w334:refnum<file>, error out=w333:errorcluster)  [unwired: 1 in]
                          n247 = Write to Text File(file (use dialog)=w334, text=w328, error in=w333) -> (refnum out=w338:refnum<file>, error out=w339:errorcluster)  [unwired: 2 out]
                          n248 = Close File(refnum=w338, error in=w339) -> (path=w330:path, error out=w331:errorcluster)
                          n249 = call <vilib>:"Simple Error Handler.vi"("error in (no error)"=w331) -> ("error out"=w329:errorcluster)  [unwired: 1 in, 7 out]
                        }
                        frame #1 {
                          n250 = local write "Estagio auto"(7 ("Estagio auto")) -> ()
                          n251 = local write "teste slope"(0 ("teste slope")) -> ()
                          n252 = local write "Pit 2"(TRUE ("ZPit")) -> ()
                          n253 = local write "N fit"("N fit patamar") -> ()
                          n254 = Wait (ms)(milliseconds to wait=u32 500) -> ()  [unwired: 1 out]
                          n255 = Read from Text File(file (use dialog)=w347, count=-1 ("Count  3"), error in=w346) -> (refnum out=w348:refnum<file>, text=w352:string, error out=w349:errorcluster)  [unwired: 1 in, 1 out]
                          n256 = local write "String 3"(w352) -> ()
                          n257 = Close File(refnum=w348, error in=w349) -> (error out=w350:errorcluster)  [unwired: 1 out]
                          n258 = call <vilib>:"Simple Error Handler.vi"("error in (no error)"=w350) -> ()  [unwired: 1 in, 8 out]
                          n259 = local write "String"("abrir valvula entrada camara" ("String")) -> ()
                        }
                      }
                    }
                  }
                }
                frame 7 {
                  n260 = flat-sequence {
                    tunnel: w356 -> [w368]
                    tunnel: w355 -> [w367]
                    tunnel: w354 -> [w366]
                    frame #0 {
                      w381 = "\t"
                      w387 = i16 4 ("precision (6)")
                      n261 = Number To Fractional String(number=w367, precision (6)=w387) -> (F-format string=w382:string)  [unwired: 2 in]
                      n262 = Number To Fractional String(number=w366, precision (6)=w387) -> (F-format string=w380:string)  [unwired: 2 in]
                      n263 = Get Date/Time String(date format (0)=enum16{"short", "long", "abbreviated"}."short", want seconds? (F)=TRUE) -> (date string=w384:string, time string=w383:string)  [unwired: 1 in]
                      n264 = Open/Create/Replace File(file path (use dialog)=w368, operation (0:open)=T2."open") -> (refnum out=w376:refnum<file>, error out=w369:errorcluster)  [unwired: 2 in, 3 out]
                      n265 = Concatenate Strings(w384, w381, w383, w381, w382, w381, w380, "\r\n") -> (w370:string)
                      n266 = Set File Position(refnum=w376, from (0:start)=enum16{"start", "end", "current"}."end", error in=w369) -> (refnum out=w374:refnum<file>, error out=w373:errorcluster)  [unwired: 1 in]
                      n267 = Write to Text File(file (use dialog)=w374, text=w370, error in=w373) -> (refnum out=w377:refnum<file>, error out=w378:errorcluster)  [unwired: 2 out]
                      n268 = Close File(refnum=w377, error in=w378) -> (error out=w371:errorcluster)  [unwired: 1 out]
                      n269 = call <vilib>:"Simple Error Handler.vi"("error in (no error)"=w371) -> ()  [unwired: 1 in, 8 out]
                    }
                  }
                  n270 = property on="Contador" class="DigNum (strict)"() -> ("Value"=w364:i32)  [unwired: 2 in, 2 out]
                  n271 = property on="N fit patamar" class="DigNum (strict)"() -> ("Value"=w353:i32)  [unwired: 2 in, 2 out]
                  n272 = Increment(x=w364) -> (x+1=w363:i32)
                  n273 = Equal?(x=w363, y=w353) -> (x = y?=w365:bool)
                  n274 = case shown="True" w365 {
                    tunnel: [FALSE w392] -> w362
                    tunnel: [_ w391] -> w361
                    frame False {
                    }
                    frame True {
                      n275 = property on="P slope" class="DigNum (strict)"() -> ("Value"=w394:dbl)  [unwired: 2 in, 2 out]
                      n276 = Absolute Value(x=w394) -> (abs(x)=w393:dbl)
                      n277 = Less Or Equal?(x=w393, y="STOP Slope") -> (x <= y?=w392:bool)
                      n278 = case shown="True" w392 {
                        tunnel: [_ w396] -> w391
                        frame False {
                        }
                        frame True {
                          n279 = property on="teste slope" class="DigNum (strict)"() -> ("Value"=w397:i32)  [unwired: 2 in, 2 out]
                          n280 = local write "Estagio auto"(7 ("Estagio auto")) -> ()
                          n281 = Increment(x=w397) -> (x+1=w396:i32)
                          "teste slope" <- w396
                        }
                      }
                    }
                  }
                  n282 = Greater Or Equal?(x=w361, y=5) -> (x >= y?=w359:bool)
                  n283 = And(x=w365, y=w359) -> (x .and. y?=w358:bool)
                  n284 = case shown="True" w358 {
                    frame False {
                    }
                    frame True {
                      n285 = flat-sequence {
                        frame #0 {
                          n286 = Wait (ms)(milliseconds to wait=u32 500) -> ()  [unwired: 1 out]
                          n287 = local write "N fit"(100 ("N fit")) -> ()
                        }
                        frame #1 {
                          n288 = local write "Estagio auto"(8 ("Estagio auto")) -> ()
                        }
                      }
                    }
                  }
                  n289 = case shown="True" w358 {
                    tunnel: [TRUE ("Boolean") FALSE ("Boolean")] -> w357
                    frame False {
                    }
                    frame True {
                    }
                  }
                  n290 = case shown="False" w362 {
                    tunnel: w357 -> [_ w413]
                    frame False {
                      w411 = T4 3 items=["no dialog", "OK message", "continue or stop message", "OK message + warnings", "continue/stop + warnings"] ("type of dialog (OK msg:1)")
                      w407 = TRUE ("Boolean")
                      n291 = Wait (ms)(milliseconds to wait="patamar milliseconds to wait") -> ()  [unwired: 1 out]
                      n292 = call-poly <vilib>:"DAQmx Create Virtual Channel.vi"("lines"=tag "Dev1/port0/line3") -> ("task out"=w400:refnum<k21>, "error out"=w401:errorcluster)  [unwired: 13 in]
                      n293 = call <vilib>:"DAQmx Start Task.vi"("task/channels in"=w400, "error in"=w401) -> ("task out"=w402:refnum<k21>, "error out"=w403:errorcluster)  [unwired: 12 in]
                      n294 = local write "Câmara 2"(w407) -> ()
                      n295 = case shown="True" w407 {
                        frame False {
                        }
                        frame True {
                          n296 = property on="Vol Ref 3" class="Slide (strict)"() -> ("Value"=w412:dbl)  [unwired: 2 in, 2 out]
                          n297 = local write "Camara 2"(w412) -> ()
                        }
                      }
                      n298 = call-poly <vilib>:"DAQmx Write.vi"("task/channels in"=w402, "data"=w407, "error in"=w403) -> ("task out"=w408:refnum<k21>, "error out"=w409:errorcluster)  [unwired: 10 in, 1 out]
                      n299 = call <vilib>:"DAQmx Stop Task.vi"("task/channels in"=w408, "error in"=w409) -> ("task out"=w405:refnum<k21>, "error out"=w404:errorcluster)  [unwired: 12 in]
                      n300 = call <vilib>:"DAQmx Clear Task.vi"("task in"=w405, "error in"=w404) -> ("error out"=w410:errorcluster)  [unwired: 13 in]
                      n301 = call <vilib>:"Simple Error Handler.vi"("type of dialog (OK msg:1)"=w411, "error in (no error)"=w410) -> ()  [unwired: 3 in, 5 out]
                    }
                    frame True {
                      n302 = flat-sequence {
                        tunnel: w413 -> [w414]
                        frame #0 {
                          w416 = T4 3 items=["no dialog", "OK message", "continue or stop message", "OK message + warnings", "continue/stop + warnings"] ("type of dialog (OK msg:1)")
                          n303 = local write "Câmara 2"(w414) -> ()
                          n304 = call-poly <vilib>:"DAQmx Create Virtual Channel.vi"("lines"=tag "Dev1/port0/line3") -> ("task out"=w425:refnum<k21>, "error out"=w424:errorcluster)  [unwired: 13 in]
                          n305 = call <vilib>:"DAQmx Start Task.vi"("task/channels in"=w425, "error in"=w424) -> ("task out"=w423:refnum<k21>, "error out"=w422:errorcluster)  [unwired: 12 in]
                          n306 = call-poly <vilib>:"DAQmx Write.vi"("task/channels in"=w423, "data"=w414, "error in"=w422) -> ("task out"=w418:refnum<k21>, "error out"=w417:errorcluster)  [unwired: 10 in, 1 out]
                          n307 = call <vilib>:"DAQmx Stop Task.vi"("task/channels in"=w418, "error in"=w417) -> ("task out"=w420:refnum<k21>, "error out"=w421:errorcluster)  [unwired: 12 in]
                          n308 = call <vilib>:"DAQmx Clear Task.vi"("task in"=w420, "error in"=w421) -> ("error out"=w415:errorcluster)  [unwired: 13 in]
                          n309 = call <vilib>:"Simple Error Handler.vi"("type of dialog (OK msg:1)"=w416, "error in (no error)"=w415) -> ()  [unwired: 3 in, 5 out]
                        }
                        frame #1 {
                          n310 = Wait (ms)(milliseconds to wait=u32 2000) -> ()  [unwired: 1 out]
                        }
                      }
                    }
                  }
                }
                frame 8 {
                  n311 = property on="Contador" class="DigNum (strict)"() -> ("Value"=w431:i32)  [unwired: 2 in, 2 out]
                  n312 = Increment(x=w431) -> (x+1=w433:i32)
                  n313 = Equal?(x=w433, y=100) -> (x = y?=w430:bool)
                  n314 = case shown="True" w430 {
                    tunnel: w434 -> [_ w435]
                    frame False {
                    }
                    frame True {
                      n315 = property on="P fit" class="DigNum (strict)"() -> ("Value"=w436:dbl)  [unwired: 2 in, 2 out]
                      n316 = Number To Fractional String(number=w436, precision (6)=i16 3) -> (F-format string=w440:string)  [unwired: 2 in]
                      n317 = Concatenate Strings(w440, "\t") -> (w438:string)
                      n318 = flat-sequence {
                        tunnel: [w447] -> w442
                        tunnel: [w446] -> w441
                        tunnel: w438 -> [w445]
                        tunnel: w435 -> [w444]
                        tunnel: w442 -> [w462]
                        tunnel: w441 -> [w461]
                        frame #0 {
                          n319 = Wait (ms)(milliseconds to wait=u32 500) -> ()  [unwired: 1 out]
                          n320 = Open/Create/Replace File(file path (use dialog)=w444, operation (0:open)=T2."open") -> (refnum out=w453:refnum<file>, error out=w454:errorcluster)  [unwired: 2 in, 3 out]
                          n321 = Set File Position(refnum=w453, from (0:start)=enum16{"start", "end", "current"}."end", error in=w454) -> (refnum out=w451:refnum<file>, error out=w450:errorcluster)  [unwired: 1 in]
                          n322 = Write to Text File(file (use dialog)=w451, text=w445, error in=w450) -> (refnum out=w455:refnum<file>, error out=w456:errorcluster)  [unwired: 2 out]
                          n323 = Close File(refnum=w455, error in=w456) -> (path=w447:path, error out=w448:errorcluster)
                          n324 = call <vilib>:"Simple Error Handler.vi"("error in (no error)"=w448) -> ("error out"=w446:errorcluster)  [unwired: 1 in, 7 out]
                        }
                        frame #1 {
                          n325 = local write "Estagio auto"(9 ("Estagio auto")) -> ()
                          n326 = local write "Pf2 2"(TRUE ("ZPit")) -> ()
                          n327 = Wait (ms)(milliseconds to wait=u32 500) -> ()  [unwired: 1 out]
                          n328 = Read from Text File(file (use dialog)=w462, count=-1 ("Count  3"), error in=w461) -> (refnum out=w463:refnum<file>, text=w467:string, error out=w464:errorcluster)  [unwired: 1 in, 1 out]
                          n329 = local write "String 3"(w467) -> ()
                          n330 = Close File(refnum=w463, error in=w464) -> (error out=w465:errorcluster)  [unwired: 1 out]
                          n331 = local write "String"("abrir valvula vacuo" ("String")) -> ()
                          n332 = call <vilib>:"Simple Error Handler.vi"("error in (no error)"=w465) -> ()  [unwired: 1 in, 8 out]
                        }
                      }
                    }
                  }
                }
                frame 9 {
                  n333 = Greater?(x=w468, y=1.0) -> (0:w473:bool)
                  n334 = case shown="False" w473 {
                    tunnel: [FALSE ("Boolean") TRUE ("Boolean")] -> w471
                    frame False {
                      w493 = TRUE ("Boolean")
                      n335 = Multiply(x="ZPf2 time", y=0.0741) -> (x*y=w488:dbl)
                      n336 = Add(x=w488, y=1.9801) -> (x+y=w486:dbl)
                      n337 = local write "Vácuo 2"(w493) -> ()
                      n338 = call "Controle_vacuo.vi"("time (s) to wait vacuo"=w486, "Boolean"=w493) -> ("Vacuo"=w494:bool)  [unwired: 9 in]
                      n339 = local write "Vácuo 2"(w494) -> ()
                      n340 = local write "String"("Limpar volume referencia" ("String")) -> ()
                    }
                    frame True {
                      n341 = property on="ATM wait" class="DigNum (strict)"() -> ("Value"=w495:u32)  [unwired: 2 in, 2 out]
                      n342 = call "Controle_ATM.vi"("seconds to wait"=w495) -> ("String 2"=w498:string, "Atm"=w497:bool)  [unwired: 9 in]
                      n343 = local write "Atm 2"(w497) -> ()
                      n344 = local write "String"(w498) -> ()
                    }
                  }
                  n345 = for {
                    N: 1 -> [_]
                    tunnel: [w475] -> w470
                    tunnel: w471 -> [w475]
                    n346 = Wait (ms)(milliseconds to wait=u32 500 ("x")) -> ()  [unwired: 1 out]
                  }
                  n347 = case shown="True" w470 {
                    frame False {
                      n348 = local write "Estagio auto"(10 ("Estagio auto")) -> ()
                    }
                    frame True {
                      w484 = TRUE ("Boolean")
                      n349 = property on="ZPf2 time" class="DigNum (strict)"() -> ("Value"=w478:dbl)  [unwired: 2 in, 2 out]
                      n350 = Multiply(x=w478, y=0.0741) -> (x*y=w480:dbl)
                      n351 = local write "Estagio auto"(10 ("Estagio auto")) -> ()
                      n352 = Add(x=w480, y=1.9801) -> (x+y=w477:dbl)
                      n353 = local write "Vácuo 2"(w484) -> ()
                      n354 = call "Controle_vacuo.vi"("time (s) to wait vacuo"=w477, "Boolean"=w484) -> ("Vacuo"=w485:bool)  [unwired: 9 in]
                      n355 = local write "Vácuo 2"(w485) -> ()
                      n356 = local write "String"("Limpar volume referencia" ("String")) -> ()
                    }
                  }
                }
                frame 10 {
                  n357 = property on="Contador" class="DigNum (strict)"() -> ("Value"=w499:i32)  [unwired: 2 in, 2 out]
                  n358 = local write "String"("Ler ZPf2 e T" ("String")) -> ()
                  n359 = Increment(x=w499) -> (x+1=w502:i32)
                  n360 = Equal?(x=w502, y=100) -> (x = y?=w500:bool)
                  n361 = case shown="True" w500 {
                    frame False {
                    }
                    frame True {
                      n362 = local write "Estagio auto"(11 ("Estagio auto")) -> ()
                    }
                  }
                }
                frame 11 {
                  n363 = property on="Contador" class="DigNum (strict)"() -> ("Value"=w506:i32)  [unwired: 2 in, 2 out]
                  n364 = Increment(x=w506) -> (x+1=w508:i32)
                  n365 = Equal?(x=w508, y=100) -> (x = y?=w505:bool)
                  n366 = case shown="True" w505 {
                    tunnel: w509 -> [_ w519]
                    frame False {
                    }
                    frame True {
                      w513 = i16 3 ("precision (6)")
                      n367 = property on="P fit" class="DigNum (strict)"() -> ("Value"=w511:dbl)  [unwired: 2 in, 2 out]
                      n368 = property on="T fit" class="DigNum (strict)"() -> ("Value"=w512:dbl)  [unwired: 2 in, 2 out]
                      n369 = Number To Fractional String(number=w511, precision (6)=w513) -> (F-format string=w518:string)  [unwired: 2 in]
                      n370 = Number To Fractional String(number=w512, precision (6)=w513) -> (F-format string=w516:string)  [unwired: 2 in]
                      n371 = Concatenate Strings(w518, "\t", w516, "\r\n") -> (w514:string)
                      n372 = flat-sequence {
                        tunnel: [w527] -> w523
                        tunnel: [w526] -> w522
                        tunnel: w514 -> [w525]
                        tunnel: w519 -> [w524]
                        tunnel: w523 -> [w545]
                        tunnel: w522 -> [w544]
                        tunnel: [w537] -> w521
                        tunnel: [w539] -> w520
                        tunnel: w521 -> [w564]
                        tunnel: w520 -> [w560]
                        tunnel: [w563] -> w510
                        tunnel: w510 -> [w576]
                        frame #0 {
                          n373 = Open/Create/Replace File(file path (use dialog)=w524, operation (0:open)=T2."open") -> (refnum out=w533:refnum<file>, error out=w534:errorcluster)  [unwired: 2 in, 3 out]
                          n374 = Set File Position(refnum=w533, from (0:start)=enum16{"start", "end", "current"}."end", error in=w534) -> (refnum out=w531:refnum<file>, error out=w530:errorcluster)  [unwired: 1 in]
                          n375 = Write to Text File(file (use dialog)=w531, text=w525, error in=w530) -> (refnum out=w535:refnum<file>, error out=w536:errorcluster)  [unwired: 2 out]
                          n376 = Close File(refnum=w535, error in=w536) -> (path=w527:path, error out=w528:errorcluster)
                          n377 = call <vilib>:"Simple Error Handler.vi"("error in (no error)"=w528) -> ("error out"=w526:errorcluster)  [unwired: 1 in, 7 out]
                        }
                        frame #1 {
                          w541 = TRUE ("ZPit")
                          n378 = property on="SET" class="DigNum (strict)"() -> ("Value"=w540:i32)  [unwired: 2 in, 2 out]
                          n379 = Wait (ms)(milliseconds to wait=u32 500) -> ()  [unwired: 1 out]
                          n380 = local write "T 2"(w541) -> ()
                          n381 = local write "ZPf2 2"(w541) -> ()
                          n382 = Read from Text File(file (use dialog)=w545, count=-1 ("Count  3"), error in=w544) -> (refnum out=w546:refnum<file>, text=w550:string, error out=w547:errorcluster)  [unwired: 1 in, 1 out]
                          n383 = Increment(x=w540) -> (x+1=w537:i32)
                          n384 = local write "String 3"(w550) -> ()
                          n385 = Close File(refnum=w546, error in=w547) -> (error out=w548:errorcluster)  [unwired: 1 out]
                          n386 = call <vilib>:"Simple Error Handler.vi"("error in (no error)"=w548) -> ()  [unwired: 1 in, 8 out]
                          n387 = case shown="False" "Boolean" {
                            selector: "Boolean" -> [w552 w556]
                            tunnel: [w553 w559] -> w539
                            tunnel: w537 -> [w554 _]
                            frame False {
                              n388 = Not(x=w552) -> (.not. x?=→"Boolean 3":bool)
                              n389 = Index Array(array="Array", index=w554) -> (element=w553:dbl)
                            }
                            frame True {
                              n390 = property on="Set P auto" class="DigNum (strict)"() -> ("Value"=w557:dbl)  [unwired: 2 in, 2 out]
                              n391 = Add(x="Step P", y=w557) -> (x+y=w559:dbl)
                              "Boolean 2" <- w556
                            }
                          }
                          n392 = local write "String"("abrir valvula entrada gas" ("String")) -> ()
                        }
                        frame #2 {
                          n393 = local write "SET"(w564) -> ()
                          n394 = Greater?(x=w560, y="P_max") -> (0:w561:bool)
                          n395 = case shown="True" w561 {
                            tunnel: [w565 w566] -> w563
                            tunnel: "P_max" -> [_ w566]
                            tunnel: w560 -> [w565 _]
                            frame False {
                            }
                            frame True {
                            }
                          }
                        }
                        frame #3 {
                          n396 = local write "Set P auto"(w576) -> ()
                          n397 = property on="Camara 2" class="Slide (strict)"() -> ("Value"=w575:dbl)  [unwired: 2 in, 2 out]
                          n398 = Greater?(x=w575, y="P_max camara") -> (0:w573:bool)
                          n399 = property on="Carga" class="Bool (strict)"() -> ("Value"=w572:bool)  [unwired: 2 in, 2 out]
                          n400 = property on="Desc SET" class="DigNum (strict)"() -> ("Value"=w568:i32)  [unwired: 2 in, 2 out]
                          n401 = And(x=w573, y=w572) -> (x .and. y?=w570:bool)
                          n402 = Greater Than 0?(x=w568) -> (x > 0?=w567:bool)
                          n403 = case shown="False" w567 {
                            tunnel: w570 -> [w577 _]
                            tunnel: [w577 TRUE] -> w569
                            frame False {
                            }
                            frame True {
                            }
                          }
                          n404 = case shown="True" w569 {
                            tunnel: [5 ("N fit") 100 ("N fit")] -> w571
                            frame False {
                              n405 = local write "Estagio auto"(0 ("Estagio auto")) -> ()
                              "Carga" <- TRUE
                              "Descarga" <- FALSE
                            }
                            frame True {
                              n406 = local write "teste slope"(0 ("teste slope")) -> ()
                              n407 = local write "Carga"(FALSE ("Carga")) -> ()
                              n408 = local write "Descarga"(TRUE ("Descarga")) -> ()
                              n409 = local write "Estagio auto"(12 ("Estagio auto")) -> ()
                            }
                          }
                          n410 = local write "N fit"(w571) -> ()
                        }
                      }
                    }
                  }
                }
                frame 12 {
                  w592 = "\t"
                  n411 = property on="SET" class="DigNum (strict)"() -> ("Value"=w596:i32)  [unwired: 2 in, 2 out]
                  n412 = Number To Decimal String(number=w596) -> (decimal integer string=w599:string)  [unwired: 1 in]
                  n413 = Number To Fractional String(number=0.0, precision (6)=i16 3) -> (F-format string=w593:string)  [unwired: 2 in]
                  n414 = Concatenate Strings(w599, w592, w593, w592, w593, w592) -> (w598:string)
                  n415 = flat-sequence {
                    tunnel: w595 -> [w604]
                    tunnel: w598 -> [w605]
                    tunnel: [w605] -> w591
                    tunnel: [w604] -> w590
                    tunnel: [w609] -> w601
                    tunnel: [w608] -> w600
                    tunnel: w591 -> [w607]
                    tunnel: w590 -> [w606]
                    tunnel: [w606] -> w589
                    tunnel: w601 -> [w625]
                    tunnel: w600 -> [w624]
                    tunnel: w589 -> [w619]
                    tunnel: [w619] -> w588
                    tunnel: w588 -> [w631]
                    frame #0 {
                      w603 = FALSE ("ZPit 2")
                      n416 = Wait (ms)(milliseconds to wait=u32 1000) -> ()  [unwired: 1 out]
                      n417 = local write "ZPit 2"(w603) -> ()
                      n418 = local write "Pit 2"(w603) -> ()
                      n419 = local write "Pf2 2"(w603) -> ()
                      n420 = local write "ZPf2 2"(w603) -> ()
                      n421 = local write "T 2"(w603) -> ()
                    }
                    frame #1 {
                      n422 = Open/Create/Replace File(file path (use dialog)=w606, operation (0:open)=T2."open") -> (refnum out=w615:refnum<file>, error out=w616:errorcluster)  [unwired: 2 in, 3 out]
                      n423 = Set File Position(refnum=w615, from (0:start)=enum16{"start", "end", "current"}."end", error in=w616) -> (refnum out=w613:refnum<file>, error out=w612:errorcluster)  [unwired: 1 in]
                      n424 = Write to Text File(file (use dialog)=w613, text=w607, error in=w612) -> (refnum out=w617:refnum<file>, error out=w618:errorcluster)  [unwired: 2 out]
                      n425 = Close File(refnum=w617, error in=w618) -> (path=w609:path, error out=w610:errorcluster)
                      n426 = call <vilib>:"Simple Error Handler.vi"("error in (no error)"=w610) -> ("error out"=w608:errorcluster)  [unwired: 1 in, 7 out]
                    }
                    frame #2 {
                      w620 = TRUE ("ZPit")
                      n427 = local write "Estagio auto"(7 ("Estagio auto")) -> ()
                      n428 = Wait (ms)(milliseconds to wait=u32 500) -> ()  [unwired: 1 out]
                      n429 = local write "ZPit 2"(w620) -> ()
                      n430 = local write "Pit 2"(w620) -> ()
                      n431 = Read from Text File(file (use dialog)=w625, count=-1 ("Count  3"), error in=w624) -> (refnum out=w626:refnum<file>, text=w630:string, error out=w627:errorcluster)  [unwired: 1 in, 1 out]
                      n432 = local write "String 3"(w630) -> ()
                      n433 = Close File(refnum=w626, error in=w627) -> (error out=w628:errorcluster)  [unwired: 1 out]
                      n434 = local write "String"("abrir valvula camara" ("String")) -> ()
                      n435 = call <vilib>:"Simple Error Handler.vi"("error in (no error)"=w628) -> ()  [unwired: 1 in, 8 out]
                    }
                    frame #3 {
                      n436 = property on="Camara 2" class="Slide (strict)"() -> ("Value"=w638:dbl)  [unwired: 2 in, 2 out]
                      n437 = property on="Efetuados" class="DigNum (strict)"() -> ("Value"=w635:dbl)  [unwired: 2 in, 2 out]
                      n438 = Less?(x="Ciclos", y=w635) -> (x < y?=w634:bool)
                      n439 = Less?(x=w638, y="P_min descarga") -> (x < y?=w633:bool)
                      n440 = case shown="True" w633 {
                        tunnel: w635 -> [_ w655]
                        tunnel: w631 -> [_ w644]
                        frame False {
                        }
                        frame True {
                          w642 = "\r\n"
                          n441 = Increment(x=w655) -> (x+1=→"Efetuados":dbl)
                          n442 = local write "Estagio auto"(0 ("Estagio auto")) -> ()
                          n443 = local write "SET"(0 ("SET")) -> ()
                          n444 = local write "Set P auto"(0.5 ("Set P auto")) -> ()
                          n445 = Open/Create/Replace File(file path (use dialog)=w644, operation (0:open)=T2."open") -> (refnum out=w650:refnum<file>, error out=w651:errorcluster)  [unwired: 2 in, 3 out]
                          n446 = Concatenate Strings(w642, ">>>>>>>>>>>>>>" ("string"), w642, w642) -> (w641:string)
                          n447 = Set File Position(refnum=w650, from (0:start)=enum16{"start", "end", "current"}."end", error in=w651) -> (refnum out=w648:refnum<file>, error out=w647:errorcluster)  [unwired: 1 in]
                          n448 = Write to Text File(file (use dialog)=w648, text=w641, error in=w647) -> (refnum out=w652:refnum<file>, error out=w653:errorcluster)  [unwired: 2 out]
                          n449 = Close File(refnum=w652, error in=w653) -> (error out=w645:errorcluster)  [unwired: 1 out]
                          n450 = call <vilib>:"Simple Error Handler.vi"("error in (no error)"=w645) -> ()  [unwired: 1 in, 8 out]
                        }
                      }
                      n451 = And(x=w633, y=w634) -> (x .and. y?=w632:bool)
                      n452 = case shown="True" w632 {
                        frame False {
                          n453 = local write "FIM"(FALSE ("FIM")) -> ()
                        }
                        frame True {
                          w660 = 1 ("N fit")
                          n454 = local write "Auto Ctrl"(FALSE ("Auto Ctrl")) -> ()
                          n455 = local write "N fit"(w660) -> ()
                          n456 = local write "N to fit"(w660) -> ()
                          "FIM" <- TRUE ("stop")
                        }
                      }
                    }
                    frame #4 {
                      w663 = TRUE ("data")
                      w665 = T4 3 items=["no dialog", "OK message", "continue or stop message", "OK message + warnings", "continue/stop + warnings"] ("type of dialog (OK msg:1)")
                      n457 = property on="Desc SET" class="DigNum (strict)"() -> ("Value"=w661:i32)  [unwired: 2 in, 2 out]
                      n458 = Increment(x=w661) -> (x+1=→"Desc SET":i32)
                      n459 = call-poly <vilib>:"DAQmx Create Virtual Channel.vi"("lines"=tag "Dev1/port0/line3") -> ("task out"=w674:refnum<k21>, "error out"=w673:errorcluster)  [unwired: 13 in]
                      n460 = call <vilib>:"DAQmx Start Task.vi"("task/channels in"=w674, "error in"=w673) -> ("task out"=w672:refnum<k21>, "error out"=w671:errorcluster)  [unwired: 12 in]
                      n461 = local write "Câmara 2"(w663) -> ()
                      n462 = call-poly <vilib>:"DAQmx Write.vi"("task/channels in"=w672, "data"=w663, "error in"=w671) -> ("task out"=w667:refnum<k21>, "error out"=w666:errorcluster)  [unwired: 10 in, 1 out]
                      n463 = call <vilib>:"DAQmx Stop Task.vi"("task/channels in"=w667, "error in"=w666) -> ("task out"=w669:refnum<k21>, "error out"=w670:errorcluster)  [unwired: 12 in]
                      n464 = call <vilib>:"DAQmx Clear Task.vi"("task in"=w669, "error in"=w670) -> ("error out"=w664:errorcluster)  [unwired: 13 in]
                      n465 = call <vilib>:"Simple Error Handler.vi"("type of dialog (OK msg:1)"=w665, "error in (no error)"=w664) -> ()  [unwired: 3 in, 5 out]
                    }
                  }
                }
              }
            }
          }
          n466 = Index Array(array=w58, index=w56) -> (element=w55:dbl)
          n467 = Index Array(array=w57, index=w56) -> (element=w54:dbl)
          n468 = Bundle("Real 2D Array"=w61, "Best Polynomial Fit"=w62) -> (w59:T5)  [unwired: 1 in]
          n469 = Bundle("Real 2D Array"=w61, "Best Linear Fit"=w73) -> (w72:T6)  [unwired: 1 in]
          n470 = Bundle("Real 2D Array"=w61, "Real 2D Array"=w64) -> (w71:T7)  [unwired: 1 in]
          n471 = Bundle("Real 2D Array"=w61, "Best Polynomial Fit"=w63) -> (w60:T5)  [unwired: 1 in]
          n472 = Bundle("Real 2D Array"=w61, "Best Linear Fit"=w68) -> (w69:T6)  [unwired: 1 in]
          n473 = Bundle("Real 2D Array"=w61, "Real 2D Array"=w65) -> (w70:T7)  [unwired: 1 in]
          n474 = case shown="True" w53 {
            tunnel: w55 -> [_ w677]
            tunnel: w54 -> [_ w676]
            tunnel: w48 -> [_ w675]
            frame False {
            }
            frame True {
              "P fit" <- w677
              "T fit" <- w676
              "P slope" <- w675
            }
          }
          n475 = Build Array(w71, w72, w59) -> (→"Linear T":T8)
          n476 = Build Array(w70, w69, w60) -> (→"Linear P":T8)
          "Contador" <- w52
        }
        n477 = local write "time subarray"(dbl[] [0.0, 1.0] ("subarray")) -> ()
        n478 = local write "T subarray 3"(dbl[] [0.0, 1.0] ("subarray")) -> ()
        n479 = local write "P subarray 2"(dbl[] [0.0, 1.0] ("subarray")) -> ()
        n480 = local write "P T  index 2"(0 ("P T  index")) -> ()
      }
    }
    n481 = case shown="True" "Manual Ctrl" {
      frame False {
      }
      frame True {
        w762 = 0 ("polynomial order")
        n482 = for {
          N: "N to fit" -> [_]
          tunnel: [w828] -> w753 mode=indexing
          tunnel: [w833] -> w752 mode=indexing
          tunnel: [w833] -> w760 mode=indexing
          tunnel: [w826] -> w761 mode=indexing
          i -> [w833]
          n483 = call "Read P T.vi"() -> ("P Set 2 Output 2"=w834:dbl, "T Set 2 Output"=w826:dbl)  [unwired: 4 in, 6 out]
          n484 = case shown="False" "Clear" {
            frame False {
            }
            frame True {
              n485 = property on="P-manual" class="WFChart (strict)"("History Data"=dynamicdata[] []) -> ()  [unwired: 2 in, 2 out]
            }
          }
          n486 = case shown="True" "Câmara" {
            frame False {
            }
            frame True {
              n487 = property on="Vol Ref" class="Slide (strict)"() -> ("Value"=w877:dbl)  [unwired: 2 in, 2 out]
              n488 = local write "Camara"(w877) -> ()
            }
          }
          n489 = case shown="True" "Guardar\nCinetica" {
            frame False {
            }
            frame True {
              n490 = feedback #1() -> (w836:bool)  [unwired: 1 in]
              "x >= y?" <- w836
              n491 = case shown="True" w836 {
                frame False {
                }
                frame True {
                  n492 = flat-sequence {
                    tunnel: [w846] -> w841
                    tunnel: [w845] -> w840
                    tunnel: w841 -> [w867]
                    tunnel: w840 -> [w866]
                    frame #0 {
                      w859 = "\t"
                      w865 = i16 3 ("precision (6)")
                      n493 = property on="T cinetica mean 2" class="DigNum (strict)"() -> ("Value"=w842:dbl)  [unwired: 2 in, 2 out]
                      n494 = property on="path 2_cinetica" class="Path"() -> ("Value"=w844:path)  [unwired: 2 in, 2 out]
                      n495 = property on="P cinetica mean" class="DigNum (strict)"() -> ("Value"=w843:dbl)  [unwired: 2 in, 2 out]
                      n496 = Number To Fractional String(number=w843, precision (6)=w865) -> (F-format string=w860:string)  [unwired: 2 in]
                      n497 = Number To Fractional String(number=w842, precision (6)=w865) -> (F-format string=w858:string)  [unwired: 2 in]
                      n498 = Get Date/Time String(date format (0)=enum16{"short", "long", "abbreviated"}."short", want seconds? (F)=TRUE) -> (date string=w862:string, time string=w861:string)  [unwired: 1 in]
                      n499 = Open/Create/Replace File(file path (use dialog)=w844, operation (0:open)=T2."open") -> (refnum out=w853:refnum<file>, error out=w854:errorcluster)  [unwired: 2 in, 3 out]
                      n500 = Concatenate Strings(w862, w859, w861, w859, w860, w859, w858, "\r\n") -> (w847:string)
                      n501 = Set File Position(refnum=w853, from (0:start)=enum16{"start", "end", "current"}."end", error in=w854) -> (refnum out=w851:refnum<file>, error out=w850:errorcluster)  [unwired: 1 in]
                      n502 = Write to Text File(file (use dialog)=w851, text=w847, error in=w850) -> (refnum out=w855:refnum<file>, error out=w856:errorcluster)  [unwired: 2 out]
                      n503 = Close File(refnum=w855, error in=w856) -> (path=w846:path, error out=w848:errorcluster)
                      n504 = call <vilib>:"Simple Error Handler.vi"("error in (no error)"=w848) -> ("error out"=w845:errorcluster)  [unwired: 1 in, 7 out]
                    }
                    frame #1 {
                      n505 = Read from Text File(file (use dialog)=w867, count=-1 ("Count  3"), error in=w866) -> (refnum out=w868:refnum<file>, text=w872:string, error out=w869:errorcluster)  [unwired: 1 in, 1 out]
                      n506 = local write "String_cinetica"(w872) -> ()
                      n507 = Close File(refnum=w868, error in=w869) -> (error out=w870:errorcluster)  [unwired: 1 out]
                      n508 = call <vilib>:"Simple Error Handler.vi"("error in (no error)"=w870) -> ()  [unwired: 1 in, 8 out]
                    }
                    frame #2 {
                      n509 = local write "P T  index"(0 ("P T  index")) -> ()
                      n510 = local write "P subarray"(dbl[] [0.0, 1.0] ("subarray")) -> ()
                      n511 = local write "T subarray 2"(dbl[] [0.0, 1.0] ("subarray")) -> ()
                    }
                  }
                }
              }
              n512 = call "Elapsed Time"("Reset"=w836) -> ("Elapsed Time (s)"=w838:dbl)  [unwired: 11 in, 7 out]
              "Elapsed Time (sec)" <- w838
              n513 = Greater Or Equal?(x=w838, y="seconds") -> (x >= y?=w839:bool)
              n514 = feedback-in #1(w839) -> ()
            }
          }
          n515 = Multiply(x=w834, y=10.0) -> (x*y=w828:dbl)
          n516 = local write "Vol Ref"(w828) -> ()
          n517 = stacked-sequence {
            tunnel: "Entrada Gás" -> [w908 _ _ _]
            tunnel: "Vácuo" -> [_ w920 _ _]
            tunnel: "Câmara" -> [_ _ w932 _]
            tunnel: "ATM" -> [_ _ _ w944]
            frame #0 {
              w913 = T4 3 items=["no dialog", "OK message", "continue or stop message", "OK message + warnings", "continue/stop + warnings"] ("type of dialog (OK msg:1)")
              n518 = property on="Entrada gás" class="Bool (strict)"("Value"=w908) -> ()  [unwired: 2 in, 2 out]
              n519 = call-poly <vilib>:"DAQmx Create Virtual Channel.vi"("lines"=tag "Dev1/port0/line1") -> ("task out"=w911:refnum<k21>, "error out"=w912:errorcluster)  [unwired: 13 in]
              n520 = call <vilib>:"DAQmx Start Task.vi"("task/channels in"=w911, "error in"=w912) -> ("task out"=w914:refnum<k21>, "error out"=w915:errorcluster)  [unwired: 12 in]
              n521 = call-poly <vilib>:"DAQmx Write.vi"("task/channels in"=w914, "data"=w908, "error in"=w915) -> ("task out"=w919:refnum<k21>, "error out"=w916:errorcluster)  [unwired: 10 in, 1 out]
              n522 = call <vilib>:"DAQmx Stop Task.vi"("task/channels in"=w919, "error in"=w916) -> ("task out"=w918:refnum<k21>, "error out"=w917:errorcluster)  [unwired: 12 in]
              n523 = call <vilib>:"DAQmx Clear Task.vi"("task in"=w918, "error in"=w917) -> ("error out"=w910:errorcluster)  [unwired: 13 in]
              n524 = call <vilib>:"Simple Error Handler.vi"("type of dialog (OK msg:1)"=w913, "error in (no error)"=w910) -> ()  [unwired: 3 in, 5 out]
            }
            frame #1 {
              w925 = T4 3 items=["no dialog", "OK message", "continue or stop message", "OK message + warnings", "continue/stop + warnings"] ("type of dialog (OK msg:1)")
              n525 = property on="Vácuo" class="Bool (strict)"("Value"=w920) -> ()  [unwired: 2 in, 2 out]
              n526 = call-poly <vilib>:"DAQmx Create Virtual Channel.vi"("lines"=tag "Dev1/port0/line2") -> ("task out"=w923:refnum<k21>, "error out"=w924:errorcluster)  [unwired: 13 in]
              n527 = call <vilib>:"DAQmx Start Task.vi"("task/channels in"=w923, "error in"=w924) -> ("task out"=w926:refnum<k21>, "error out"=w927:errorcluster)  [unwired: 12 in]
              n528 = call-poly <vilib>:"DAQmx Write.vi"("task/channels in"=w926, "data"=w920, "error in"=w927) -> ("task out"=w931:refnum<k21>, "error out"=w928:errorcluster)  [unwired: 10 in, 1 out]
              n529 = call <vilib>:"DAQmx Stop Task.vi"("task/channels in"=w931, "error in"=w928) -> ("task out"=w930:refnum<k21>, "error out"=w929:errorcluster)  [unwired: 12 in]
              n530 = call <vilib>:"DAQmx Clear Task.vi"("task in"=w930, "error in"=w929) -> ("error out"=w922:errorcluster)  [unwired: 13 in]
              n531 = call <vilib>:"Simple Error Handler.vi"("type of dialog (OK msg:1)"=w925, "error in (no error)"=w922) -> ()  [unwired: 3 in, 5 out]
            }
            frame #2 {
              w937 = T4 3 items=["no dialog", "OK message", "continue or stop message", "OK message + warnings", "continue/stop + warnings"] ("type of dialog (OK msg:1)")
              n532 = property on="Câmara" class="Bool (strict)"("Value"=w932) -> ()  [unwired: 2 in, 2 out]
              n533 = call-poly <vilib>:"DAQmx Create Virtual Channel.vi"("lines"=tag "Dev1/port0/line3") -> ("task out"=w935:refnum<k21>, "error out"=w936:errorcluster)  [unwired: 13 in]
              n534 = call <vilib>:"DAQmx Start Task.vi"("task/channels in"=w935, "error in"=w936) -> ("task out"=w938:refnum<k21>, "error out"=w939:errorcluster)  [unwired: 12 in]
              n535 = call-poly <vilib>:"DAQmx Write.vi"("task/channels in"=w938, "data"=w932, "error in"=w939) -> ("task out"=w943:refnum<k21>, "error out"=w940:errorcluster)  [unwired: 10 in, 1 out]
              n536 = call <vilib>:"DAQmx Stop Task.vi"("task/channels in"=w943, "error in"=w940) -> ("task out"=w942:refnum<k21>, "error out"=w941:errorcluster)  [unwired: 12 in]
              n537 = call <vilib>:"DAQmx Clear Task.vi"("task in"=w942, "error in"=w941) -> ("error out"=w934:errorcluster)  [unwired: 13 in]
              n538 = call <vilib>:"Simple Error Handler.vi"("type of dialog (OK msg:1)"=w937, "error in (no error)"=w934) -> ()  [unwired: 3 in, 5 out]
            }
            frame #3 {
              w949 = T4 3 items=["no dialog", "OK message", "continue or stop message", "OK message + warnings", "continue/stop + warnings"] ("type of dialog (OK msg:1)")
              n539 = property on="Atm" class="Bool (strict)"("Value"=w944) -> ()  [unwired: 2 in, 2 out]
              n540 = call-poly <vilib>:"DAQmx Create Virtual Channel.vi"("lines"=tag "Dev1/port0/line4") -> ("task out"=w947:refnum<k21>, "error out"=w948:errorcluster)  [unwired: 13 in]
              n541 = call <vilib>:"DAQmx Start Task.vi"("task/channels in"=w947, "error in"=w948) -> ("task out"=w950:refnum<k21>, "error out"=w951:errorcluster)  [unwired: 12 in]
              n542 = call-poly <vilib>:"DAQmx Write.vi"("task/channels in"=w950, "data"=w944, "error in"=w951) -> ("task out"=w955:refnum<k21>, "error out"=w952:errorcluster)  [unwired: 10 in, 1 out]
              n543 = call <vilib>:"DAQmx Stop Task.vi"("task/channels in"=w955, "error in"=w952) -> ("task out"=w954:refnum<k21>, "error out"=w953:errorcluster)  [unwired: 12 in]
              n544 = call <vilib>:"DAQmx Clear Task.vi"("task in"=w954, "error in"=w953) -> ("error out"=w946:errorcluster)  [unwired: 13 in]
              n545 = call <vilib>:"Simple Error Handler.vi"("type of dialog (OK msg:1)"=w949, "error in (no error)"=w946) -> ()  [unwired: 3 in, 5 out]
            }
          }
          n546 = stacked-sequence {
            tunnel: w828 -> [w900 _]
            tunnel: w826 -> [w879 _]
            frame #0 {
              w878 = 2 ("y")
              n547 = property on="P T  index" class="DigNum (strict)"() -> ("Value"=w880:i32)  [unwired: 2 in, 2 out]
              n548 = property on="P subarray" class="Arr (strict)"() -> ("Value"=w902:dbl[])  [unwired: 2 in, 2 out]
              n549 = Replace Array Subset(array=w902, new element=w900, index=w880) -> (w898:dbl[])
              n550 = property on="T subarray 2" class="Arr (strict)"() -> ("Value"=w889:dbl[])  [unwired: 2 in, 2 out]
              n551 = Replace Array Subset(array=w889, new element=w879, index=w880) -> (w886:dbl[])
              n552 = call-poly <vilib>:"Array To Matrix.vi"("Real 1D Array"=w898) -> ("Real Matrix (Column Vector)"=w905:T3)
              n553 = Matrix Size(0:w905) -> (1:w904:i32, 2:w903:i32)
              n554 = call-poly <vilib>:"Array To Matrix.vi"("Real 1D Array"=w886) -> ("Real Matrix (Column Vector)"=w892:T3)
              n555 = Matrix Size(0:w892) -> (1:w891:i32, 2:w890:i32)
              n556 = Increment(x=w904) -> (x+1=w893:i32)
              n557 = Subtract(x=w893, y=w878) -> (x-y=w894:i32)
              n558 = Resize Matrix(1:w903, 2:w893, 4:w905) -> (0:w901:T3)
              n559 = Increment(x=w891) -> (x+1=w881:i32)
              n560 = Subtract(x=w881, y=w878) -> (x-y=w882:i32)
              n561 = Resize Matrix(1:w890, 2:w881, 4:w892) -> (0:w888:T3)
              n562 = call-poly <vilib>:"Matrix To Array.vi"("Real Matrix"=w901) -> ("Real 2D Array"=w896:dbl[][])
              n563 = call-poly <vilib>:"Matrix To Array.vi"("Real Matrix"=w888) -> ("Real 2D Array"=w884:dbl[][])
              n564 = Reshape Array(w896, w893) -> (w895:dbl[])
              n565 = local write "P subarray"(w895) -> ()
              n566 = Reshape Array(w895, w894) -> (w897:dbl[])
              n567 = Reshape Array(w884, w881) -> (w883:dbl[])
              n568 = local write "T subarray 2"(w883) -> ()
              n569 = call <vilib>:"Mean.vi"("X"=w897) -> ("mean"=→"P cinetica mean":dbl)  [unwired: 1 out]
              n570 = Reshape Array(w883, w882) -> (w885:dbl[])
              n571 = call <vilib>:"Mean.vi"("X"=w885) -> ("mean"=→"T cinetica mean 2":dbl)  [unwired: 1 out]
            }
            frame #1 {
              n572 = property on="P T  index" class="DigNum (strict)"() -> ("Value"=w907:i32)  [unwired: 2 in, 2 out]
              n573 = Increment(x=w907) -> (x+1=w906:i32)
              n574 = local write "P T  index"(w906) -> ()
            }
          }
          n575 = Merge Signals(w828, w826) -> (→"P-manual":dynamicdata)
          "N" <- w833
        }
        n576 = case shown="True" "Save manual" {
          selector: "Save manual" -> [_ w767]
          frame False {
          }
          frame True {
            n577 = feedback #2() -> (w763:dbl)  [unwired: 1 in]
            n578 = Equal To 0?(x=w763) -> (x = 0?=w769:bool)
            n579 = stacked-sequence {
              tunnel: w769 -> [_ w783 _]
              tunnel: [_ w782 _] -> w765
              frame #0 {
                w780 = i16 3 ("precision (6)")
                n580 = property on="T fit" class="DigNum (strict)"() -> ("Value"=w777:dbl)  [unwired: 2 in, 2 out]
                n581 = property on="p fit" class="DigNum (strict)"() -> ("Value"=w778:dbl)  [unwired: 2 in, 2 out]
                n582 = Number To Fractional String(number=w777, precision (6)=w780) -> (F-format string=→"T string":string)  [unwired: 2 in]
                n583 = Number To Fractional String(number=w778, precision (6)=w780) -> (F-format string=→"P string":string)  [unwired: 2 in]
              }
              frame #1 {
                n584 = case shown="True" w783 {
                  tunnel: [TRUE ("y") FALSE ("y")] -> w782
                  frame False {
                    n585 = property on="path" class="Path"() -> ("Value"=w787:path)  [unwired: 2 in, 2 out]
                    n586 = property on="P string" class="Str"() -> ("Value"=w786:string)  [unwired: 2 in, 2 out]
                    n587 = Concatenate Strings(w786, "\t") -> (w784:string)
                    n588 = Open/Create/Replace File(file path (use dialog)=w787, operation (0:open)=T2."open") -> (refnum out=w791:refnum<file>, error out=w790:errorcluster)  [unwired: 2 in, 3 out]
                    n589 = Set File Position(refnum=w791, from (0:start)=enum16{"start", "end", "current"}."end", error in=w790) -> (refnum out=w793:refnum<file>, error out=w794:errorcluster)  [unwired: 1 in]
                    n590 = Write to Text File(file (use dialog)=w793, text=w784, error in=w794) -> (refnum out=w789:refnum<file>, error out=w788:errorcluster)  [unwired: 2 out]
                    n591 = Close File(refnum=w789, error in=w788) -> (error out=w796:errorcluster)  [unwired: 1 out]
                    n592 = call <vilib>:"Simple Error Handler.vi"("error in (no error)"=w796) -> ()  [unwired: 1 in, 8 out]
                  }
                  frame True {
                    n593 = property on="path" class="Path"() -> ("Value"=w803:path)  [unwired: 2 in, 2 out]
                    n594 = property on="Count SET" class="DigNum (strict)"() -> ("Value"=w799:i32)  [unwired: 2 in, 2 out]
                    n595 = Open/Create/Replace File(file path (use dialog)=w803, operation (0:open)=T2."open") -> (refnum out=w802:refnum<file>, error out=w801:errorcluster)  [unwired: 2 in, 3 out]
                    n596 = Increment(x=w799) -> (x+1=w800:i32)
                    "Set atual" <- w800
                    n597 = Number To Decimal String(number=w800) -> (decimal integer string=w805:string)  [unwired: 1 in]
                    n598 = property on="T string" class="Str"() -> ("Value"=w807:string)  [unwired: 2 in, 2 out]
                    n599 = Concatenate Strings(w807, "\r\n", w805, "\t") -> (w808:string)
                    n600 = Set File Position(refnum=w802, from (0:start)=enum16{"start", "end", "current"}."end", error in=w801) -> (refnum out=w813:refnum<file>, error out=w814:errorcluster)  [unwired: 1 in]
                    n601 = Write to Text File(file (use dialog)=w813, text=w808, error in=w814) -> (refnum out=w811:refnum<file>, error out=w810:errorcluster)  [unwired: 2 out]
                    n602 = Close File(refnum=w811, error in=w810) -> (error out=w816:errorcluster)  [unwired: 1 out]
                    n603 = call <vilib>:"Simple Error Handler.vi"("error in (no error)"=w816) -> ()  [unwired: 1 in, 8 out]
                    "T" <- TRUE ("T")
                  }
                }
              }
              frame #2 {
                n604 = property on="path" class="Path"() -> ("Value"=w818:path)  [unwired: 2 in, 2 out]
                n605 = property on="Set atual" class="DigNum (strict)"() -> ("Value"=w817:i32)  [unwired: 2 in, 2 out]
                n606 = local write "Count SET"(w817) -> ()
                n607 = Read from Text File(file (use dialog)=w818, count=-1 ("Count  3")) -> (refnum out=w820:refnum<file>, text=w819:string, error out=w821:errorcluster)  [unwired: 2 in, 1 out]
                n608 = property on="String 2" class="Str"("Value"=w819) -> ()  [unwired: 2 in, 2 out]
                n609 = Close File(refnum=w820, error in=w821) -> (error out=w823:errorcluster)  [unwired: 1 out]
                n610 = call <vilib>:"Simple Error Handler.vi"("error in (no error)"=w823) -> ()  [unwired: 1 in, 8 out]
              }
            }
            n611 = Implies(1:w765, 2:w767) -> (0:w766:bool)
            n612 = Select(t=w763, s=w766, f=5.0 ("t")) -> (s? t:f=w764:dbl)
            n613 = Decrement(x=w764) -> (x-1=w770:dbl)
            n614 = feedback-in #2(w770) -> ()
            n615 = case shown="2" w764 {
              frame 0, Default {
              }
              frame 1 {
                "ZPf2" <- TRUE ("ZPf2")
              }
              frame 2 {
                "Pf2" <- TRUE ("Pf2")
              }
              frame 3 {
                "Pit" <- TRUE ("Pit")
              }
              frame 4 {
                n616 = local write "T"(FALSE ("T")) -> ()
                "ZPit" <- TRUE ("ZPit")
              }
              frame 5 {
                w776 = FALSE
                n617 = local write "Pit"(w776) -> ()
                n618 = local write "ZPf2"(w776) -> ()
                n619 = local write "ZPit"(w776) -> ()
                n620 = local write "Pf2"(w776) -> ()
              }
            }
          }
        }
        n621 = call <vilib>:"General Polynomial Fit.vi"("Y"=w761, "polynomial order"=w762, "X"=w760) -> ("Best Polynomial Fit"=w756:dbl[], "Polynomial Coefficients"=w757:dbl[])  [unwired: 9 in, 2 out]
        "Polynomial Coefficients 2" <- w757
        n622 = call <vilib>:"General Polynomial Fit.vi"("Y"=w753, "polynomial order"=w762, "X"=w752) -> ("Best Polynomial Fit"=w749:dbl[], "Polynomial Coefficients"=w750:dbl[])  [unwired: 9 in, 2 out]
        "Polynomial Coefficients" <- w750
        n623 = Build Array(w761, w756) -> (→"Linear Model Graph 2":dbl[][])
        n624 = Build Array(w753, w749) -> (→"Linear Model Graph":dbl[][])
        n625 = Index Array(array=w757, index=0) -> (element=→"T fit":dbl)
        n626 = Index Array(array=w750, index=0) -> (element=→"p fit":dbl)
      }
    }
    n627 = case shown="True" "Open Button 2" {
      frame False {
      }
      frame True {
        n628 = property on="Sample name" class="Str"() -> ("Value"=w726:string)  [unwired: 2 in, 2 out]
        n629 = property on="File name" class="Str"() -> ("Value"=w727:string)  [unwired: 2 in, 2 out]
        n630 = property on="Nota" class="Str"() -> ("Value"=w725:string)  [unwired: 2 in, 2 out]
        n631 = call "Open file.vi"("Nota 01"=w725, "Sample name"=w726, "File name"=w727) -> ("path open old"=w724:path)  [unwired: 8 in]
        n632 = local write "path"(w724) -> ()
      }
    }
    n633 = case shown="True" "Open Button" {
      frame False {
      }
      frame True {
        n634 = flat-sequence {
          tunnel: ["Sample name"] -> w730
          tunnel: ["Nota"] -> w729
          tunnel: [w732] -> w728
          tunnel: w730 -> [w745]
          tunnel: w729 -> [w744]
          tunnel: w728 -> [w739]
          frame #0 {
            n635 = local write "Count SET"(0 ("Count SET")) -> ()
            n636 = local write "Set atual"(0 ("Count  3")) -> ()
            n637 = call "File_data_new.vi"("Nota 01"="Nota", "Sample name"="Sample name", "File name"="File name") -> ("path"=w732:path)  [unwired: 8 in]
            "path" <- w732
          }
          frame #1 {
            w740 = FALSE
            n638 = Strip Path(path=w739) -> (stripped path=w738:path, name=w737:string)
            n639 = local write "Pf2"(w740) -> ()
            n640 = local write "ZPit"(w740) -> ()
            n641 = local write "Pit"(w740) -> ()
            n642 = local write "ZPf2"(w740) -> ()
            n643 = local write "T"(w740) -> ()
            n644 = Concatenate Strings(w737, "_cinetica" ("string")) -> (w742:string)
            n645 = call "File_data_cinetica.vi"("path in"=w738, "Nota 01"=w744, "Sample name"=w745, "File name"=w742) -> ("path"=→"path 2_cinetica":path)  [unwired: 7 in]
          }
        }
      }
    }
    n646 = property on="FIM" class="Bool (strict)"() -> ("Value"=w26:bool)  [unwired: 2 in, 2 out]
    n647 = Exclusive Or(1:w26, 2:"stop") -> (0:w28:bool)
  }
  n648 = local write "ATM wait"(u32 4 ("ATM wait")) -> ()
  n649 = local write "limpo"(0 ("limpo")) -> ()
  n650 = local write "N fit"(5 ("N fit")) -> ()
  n651 = local write "P T  index"(0 ("index")) -> ()
  n652 = local write "seconds"(2.0 ("seconds")) -> ()
  n653 = local write "N to fit"(5 ("Numeric")) -> ()
  n654 = local write "Estagio auto"(0 ("Estagio auto")) -> ()
  n655 = local write "P subarray"(dbl[] [0.0, 1.0] ("subarray")) -> ()
  n656 = local write "T subarray 2"(dbl[] [0.0, 1.0] ("subarray")) -> ()
  n657 = local write "path 2_cinetica"(path "C:/H2_Painel/painel_auto/cinetica.txt" ("path")) -> ()
  n658 = local write "path"(path "C:/H2_Painel/painel_auto/Arquivo_Padrao.txt" ("path")) -> ()
  n659 = local write "FIM"(FALSE ("FIM")) -> ()
